vi "Measurement.vi"(1 "setup":T3=enum."Show Setup", 2 "Post Process":T2, 4 "File":T4, 5 "Results file":path, 7 "Raw data file":path, 11 "Setup filename":string) -> (14 "2nd plot":cluster{"X array":dbl[], "Y array":dbl[]}[](graph), 19 "Status Out":T1)   [LabVIEW 2022 SP3]
uses:
  Anemometry Sub Vis/Globals/Meas_global.vi
  Anemometry Sub Vis/Globals/LDA_meas_global_1.vi
  Anemometry Sub Vis/Globals/Dynamic_call_global.ph.vi
  Anemometry Sub Vis/Controls/Post_Process.ctl
  Anemometry Sub Vis/Controls/Setup.ctl
  Anemometry Sub Vis/Gen Trav/Multi_Run_Status.ctl
  Anemometry Sub Vis/Globals/Trav_pos_global.vi
  Anemometry Sub Vis/Controls/Save_Data.ctl
  Anemometry Sub Vis/Acquisition/PWA/PWAtasksGLOBAL.vi
  Anemometry Sub Vis/Globals/Plug_in_data_global.vi
  Anemometry Sub Vis/Controls/Graph_Type.ctl
  ADAM Client/Sub VIs/ADAM Controls/Traverse_Level_State.ctl
  Anemometry Sub Vis/Globals/Preference_global.vi
  Anemometry Sub Vis/File/Setup_Filetype.ctl
  Anemometry Sub Vis/Controls/Inst_type.ctl
  Anemometry Sub Vis/Globals/Constants_global.vi
  Anemometry Sub Vis/Globals/Gas_management_global.vi
  Anemometry Sub Vis/Controls/Time_Trace_Cluster.ctl
  Anemometry Sub Vis/Controls/Instrument_Array.ctl
  <vilib>/Utility/miscctls.llb/LVRowAndColumnTypeDef.ctl
  Anemometry Sub Vis/Globals/LDA_global.vi
  Anemometry Sub Vis/File/File Update Cluster.ctl
  Anemometry Sub Vis/Globals/Extra_Commands_Global.vi
  Anemometry Sub Vis/CTA/CTA Calib Coeff Global.vi
  Anemometry Sub Vis/CTA/Ctls/Calibration data.ctl
panel:
  in  "PP next block":bool
  out "Pause message":string
  out "Statistics":string[][](table)
  in  "Time per Block (s)":dbl=100.0 format="%#_5f"
  out "Current Block No":i32=5 caption="Current Block"
  in  "Pause":bool
  in  "No of Blocks":i32=5
  in  "stop":bool
  out "progress":dbl(slide) scale=0.0..1.0
  in  "Tab Control":T5(tab)
  in  "Second Graph":T7={"Plot 1"=2, "Plot 2"=1, "Save graph"=0, "Plot Type"=enum."Vel histogram"} {"Save graph" items=["Do not save plot", "Save plot"]; "Plot 2" items=["Nothing", "FID4"]; "Plot 1" items=["Nothing", "FID4"]}
  in  "First Graph":T7={"Plot 1"=1, "Plot 2"=2, "Save graph"=0, "Plot Type"=enum."Velocity trace"} {"Save graph" items=["Do not save plot", "Save plot"]; "Plot 2" items=["Nothing", "FID4"]; "Plot 1" items=["Nothing", "FID4"]}
  out "First plot":cluster{"X array":dbl[], "Y array":dbl[]}[](graph)
  in  "Comments":string
  out "uv":dbl[][](graph)=[[-0.041806189081711534, -0.046435429052714985, -0.04035660097427599, -0.042187605126076694, -0.042052555599004206]]
  out "u^4":dbl[][](graph)
  out "u^3":dbl[][](graph)
  out "u^2":dbl[][](graph)=[[0.09743628875280319, 0.10575821456272283, 0.10126262927293661, 0.09890442087602569, 0.1022948212436432]]
  out "U":dbl[][](graph)=[[0.8295029456391334, 0.8915896983798417, 0.8415763502225625, 0.8394746126219594, 0.8466062785395404]]
  in  "Block average display control":cluster{"Name":string, "Include":bool}[](array[cluster])=[{"Name"="FF (C)", "Include"=FALSE}]
  out "blockDone":bool
  in  "Select Duplicate Channels":bool
  in  "Sub Block Time (s) for Spectra and Auto Corr":dbl=1.0 min=1.0 step=1.0
  in  "No of bins in histogram":i32=100
  out "Measurement time (min)":dbl=6.0 format="%.2f"
  in  "Correlate?":T8(ring)
  out "Diagnostic info":string[][](table)
  in  "No of estimates output for when saving plots":i32=200
  out "Position":T9(array[cluster]) {"Z" format="%.1f"; "Y" format="%.1f"; "X" format="%.1f"}
  out "Array U":dbl[][](array[numeric]) format="%.2e"
  out "Array u^2":dbl[][](array[numeric]) format="%.2e"
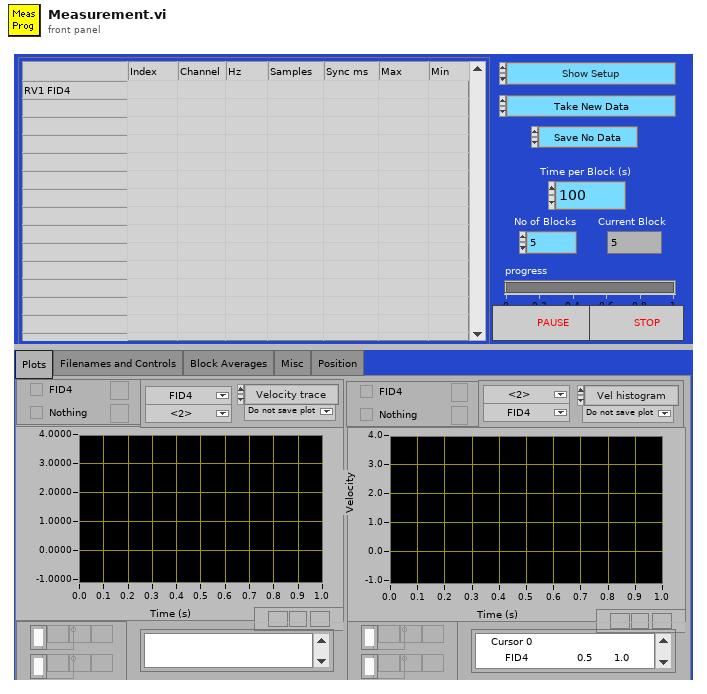
[diagram p1: front panel]
types:
  T1 = typedef "Multi_Run_Status.ctl" = enum16{"Continue", "Continue with Error", "Jump to Next Point", "Jump to Next Row", "Jump To Fall Back", "Terminate Run"}
  T2 = typedef "Post_Process.ctl" = enum16{"Take New Data", "Post Process Raw Data File"}
  T3 = typedef "Setup.ctl" = enum16{"Run Program", "Show Setup", "Save Current Setup", "Setup Front Panel"}
  T4 = typedef "Save_Data.ctl" = enum16{"Save No Data", "Save Data"}
  T5 = enum32{"Plots", "Filenames and Controls", "Block Averages", "Misc", "Position"}
  T6 = typedef "Graph_Type.ctl" = enum16{"Show no graph", "Voltage trace", "Velocity trace", "Vel histogram", "Spectrum", "f.E(f) v Log f", "Auto-Corr"}
  T7 = cluster{"Plot 1":u16, "Plot 2":u16, "Save graph":u16, "Plot Type":T6}
  T8 = enum16{"Cross correlation off", "Show correlation panel", "Correlate without activating panel"}
  T9 = cluster{"Name":string, "X":dbl, "Y":dbl, "Z":dbl}[]
  T10 = typedef "Calibration data.ctl" = cluster{"X cal.[]":dbl[], "Re cal.[]":dbl[], "a1[]":dbl[], "a2[]":dbl[], "a3[]":dbl[]}
  T11 = enum32{"Bad", "Idle", "Run top level", "Running"}
  T12 = typedef "Inst_type.ctl" = enum16{"Raw voltage", "Raw with zero offsetting", "Propeller anemometer", "Pressure Transducer", "Pitot-static tube", "Hot wire", "Cross wire 1", "Cross wire 2", "Generic Linear", "Generic Polynomial", "Generic BackPoly", "Fast FID", "Thermocouple", "Cold wire", "Pulsed Wire", "LDA Vel", "LDA Tran time", "LDA Arr time", "Microphone"}
  T13 = cluster{"Name":string, "X":dbl, "Y":dbl, "Z":dbl}
  T14 = enum32{"Invalid", "Standard", "Closed", "Hidden", "Minimized", "Maximized"}
  T15 = enum16{"Save no data", "Save data in new files", "Save data in existing files"}
  T16 = typedef "Time_Trace_Cluster.ctl" = cluster{"Weighting":dbl[], "Voltage":dbl[], "Eng Values":dbl[]}
  T17 = enum16{"Zero or one", "One", "Zero or more", "One or more"}
  T18 = typedef "Traverse_Level_State.ctl" = enum16{"Running", "Complete"}
  T19 = typedef "LVRowAndColumnTypeDef.ctl" = cluster{"Row":i32, "Column":i32}
  T20 = typedef "Instrument_Array.ctl" = enum16{"PWA", "LDA", "Analogue"}
  T21 = typedef "Setup_Filetype.ctl" = enum16{"Measurement Setups", "Calibration Setups", "General", "Results File Plotter Setups", "Speed Calib Tweaks"}
  T22 = typedef "File Update Cluster.ctl" = cluster{"File Path":path, "Rows to Add":i32[], "Extra Ch Names":string[], "Extra Ch Values":string[], "Initial Header String":string, "Separation Character":enum16{"Tab", "Comma"}}
  T23 = typedef "Analysis_info_cluster.ctl" = cluster{"Colour":u32, "Inst type":T12, "Inst name":string, "Symbol":string, "Code name":string, "Extra Info":string, "Inst Array":T20, "U":dbl, "u^2":dbl, "u^3":dbl, "u^4":dbl, "Skew_u":dbl, "Kurt_u":dbl, "Sd Error in Mean":dbl, "% u'/U":dbl, "X":dbl, "Y":dbl, "Z":dbl, "Timescale integral Estimate":dbl, "Sd Error in Variance":dbl, "Calib File":path, "Calib Constants":dbl[], "Output Position":bool, "Stats":enum16{"None", "Basic", "Full"}, "Av Sampling Rate":dbl, "Av No of Samples":dbl, "Total Meas Time (s)":dbl, "OrigChName":string, "Max value":dbl, "Min value":dbl, "Req Sample Rate Hz":dbl, "Sync Delay Time (s)":dbl, "Ch No":i16, "Device":string, "Use Latest Calib":bool, "Port":string, "Metadata Ch Names":string[], "Metadata Ch Values":string[], "Label":string, "chState":T24, "Point Drift":dbl, "inputConfig":string}
  T24 = typedef "channelState.ctl" = enum32{"No Selection", "Solo", "Mute"}
  T25 = cluster{"Insts for plotting[0]":u16, "Insts for plotting[1]":u16}
  T26 = typedef "Device ID port info.ctl" = cluster{"Ch No":i16[], "Req Sampling Rate":dbl[], "Port":string, "Index":i32[]}
  T27 = typedef "Rendezvous RefNum" = refnum<k1>
  T28 = typedef "PWA_Data.ctl" = enum16{"No PWA Data", "One Ch PWA"}
  T29 = typedef "LDA_Channel.ctl" = cluster{"Wavelength (nm)":dbl, "Vel Comp":string, "Max Velocity":dbl, "Min Velocity":dbl, "Max Record length":u16, "Signal gain (dB)":i16, "High voltage":i16, "Optics Conversion Factor":dbl, "Min Record length":u16, "Multiply Velocity by -1":bool, "Signal to Noise Ratio":string, "Validation Ratio":string, "Probe":string, "Laser":string, "BSA":string, "Lense":string, "Beam Separation (mm)":dbl, "Focal Length (mm)":dbl, "COLOUR":u32, "BSA IP":string, "Velocity Range (m/s)":dbl, "Centre Velocity (m/s)":dbl, "Unshifted mW":dbl, "Shifted mW":dbl, "Bandwidth Hz":dbl, "Req Sampling Rate Hz":dbl, "Ch":i32, "CenterFreq Hz":dbl, "Laser IP":string, "Sync Delay (s)":dbl}
  T30 = typedef "Correlation_cluster1.ctl" = cluster{"U inst":string, "uw":dbl, "u^2w":dbl, "uw^2":dbl, "uw/u'w'":dbl, "W inst":string, "uw^3":dbl, "u^3w":dbl, "u^2w^2":dbl, "Index U":i32, "Index W":i32, "Error info":string[], "Paired Sampling Rate (Hz)":dbl, "u^2 Paired":dbl, "w^2 Paired":dbl, "Time Window (ms)":dbl}
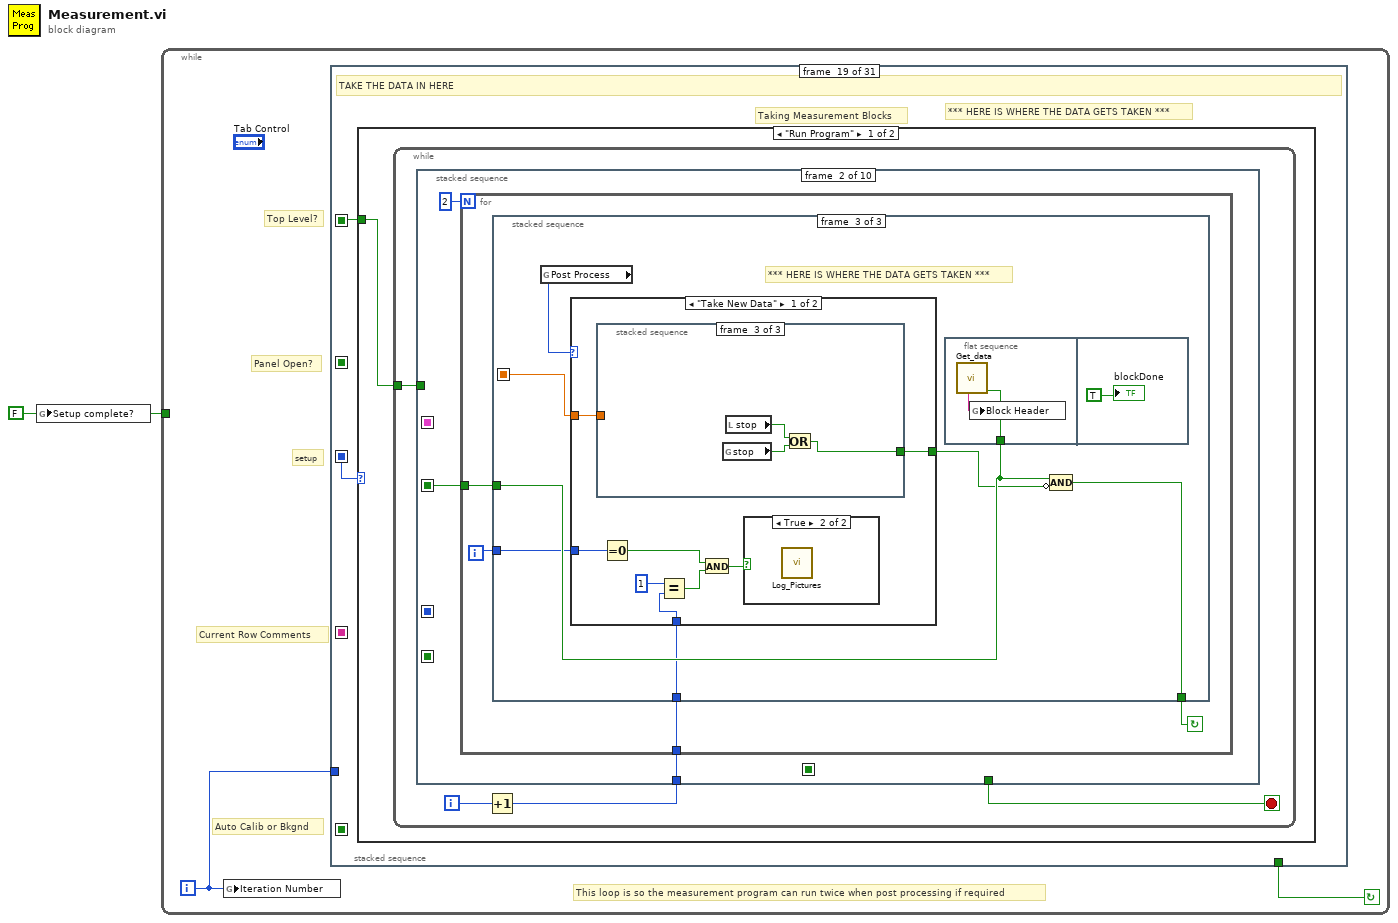
[diagram p0: block diagram]
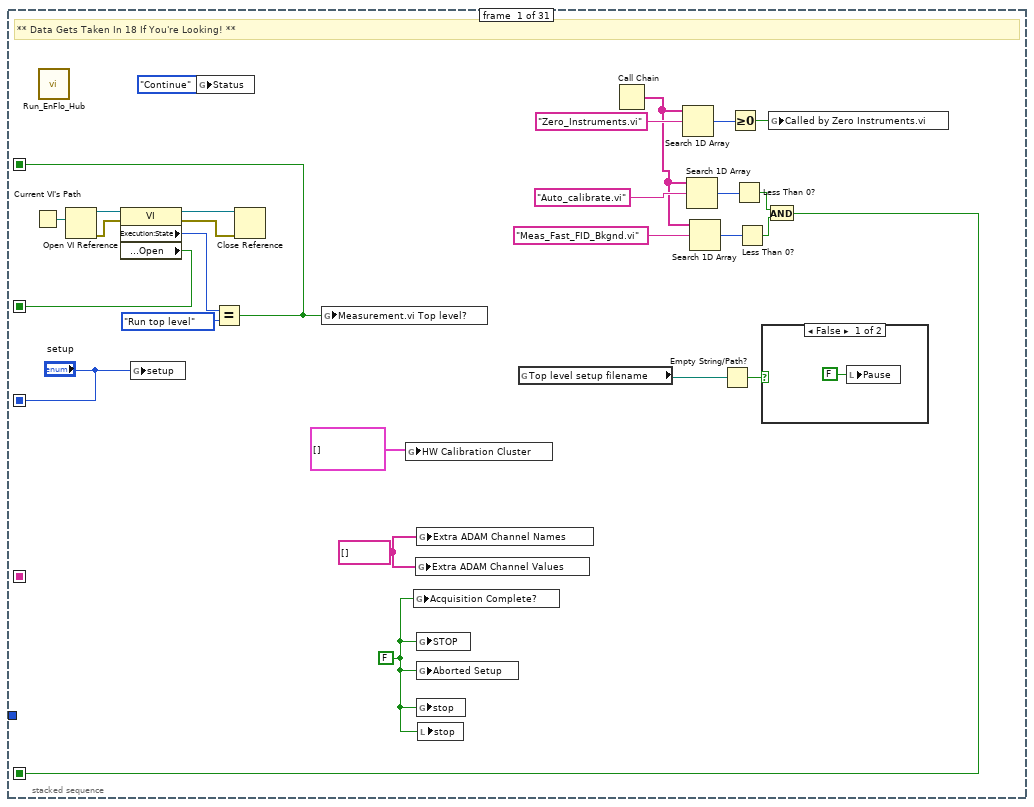
[diagram p2: hidden frame]
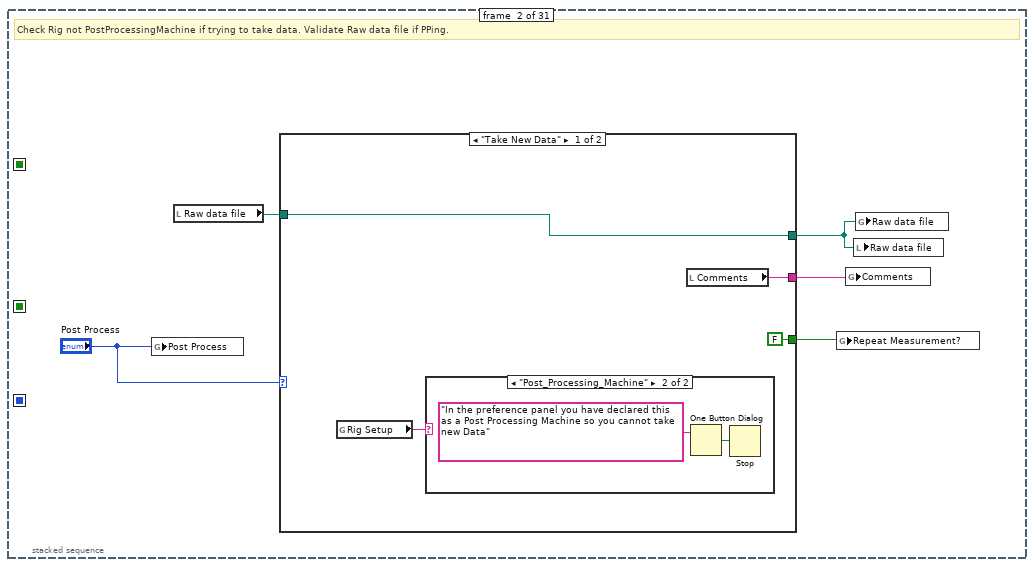
[diagram p4: hidden frame]
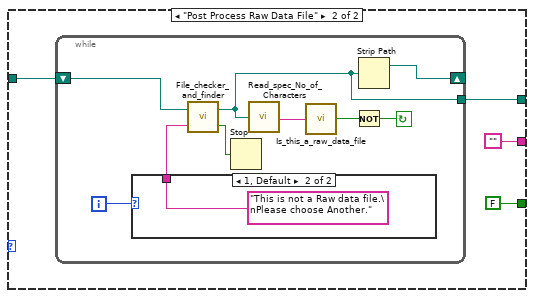
[diagram p6: hidden frame]
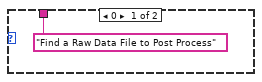
[diagram p7: hidden frame]
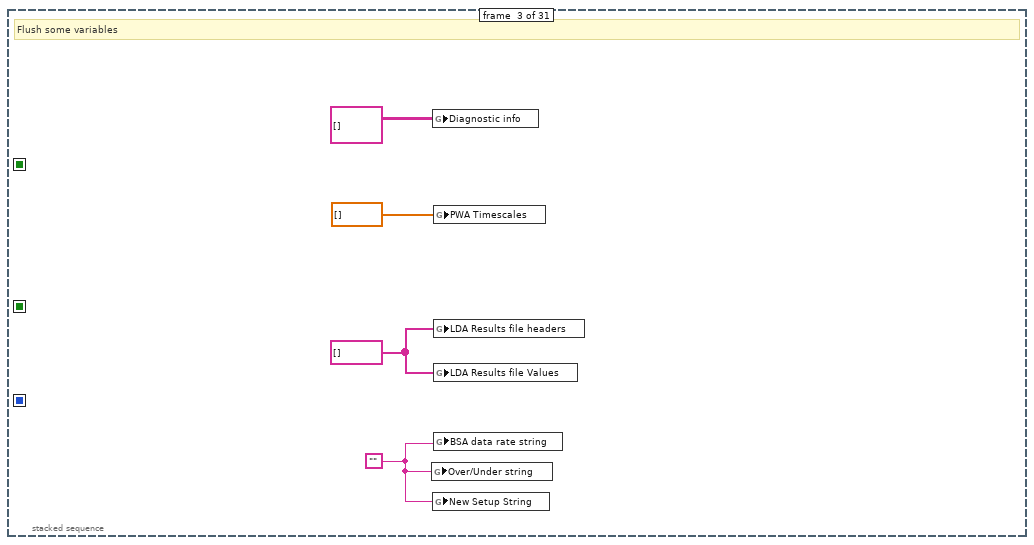
[diagram p8: hidden frame]
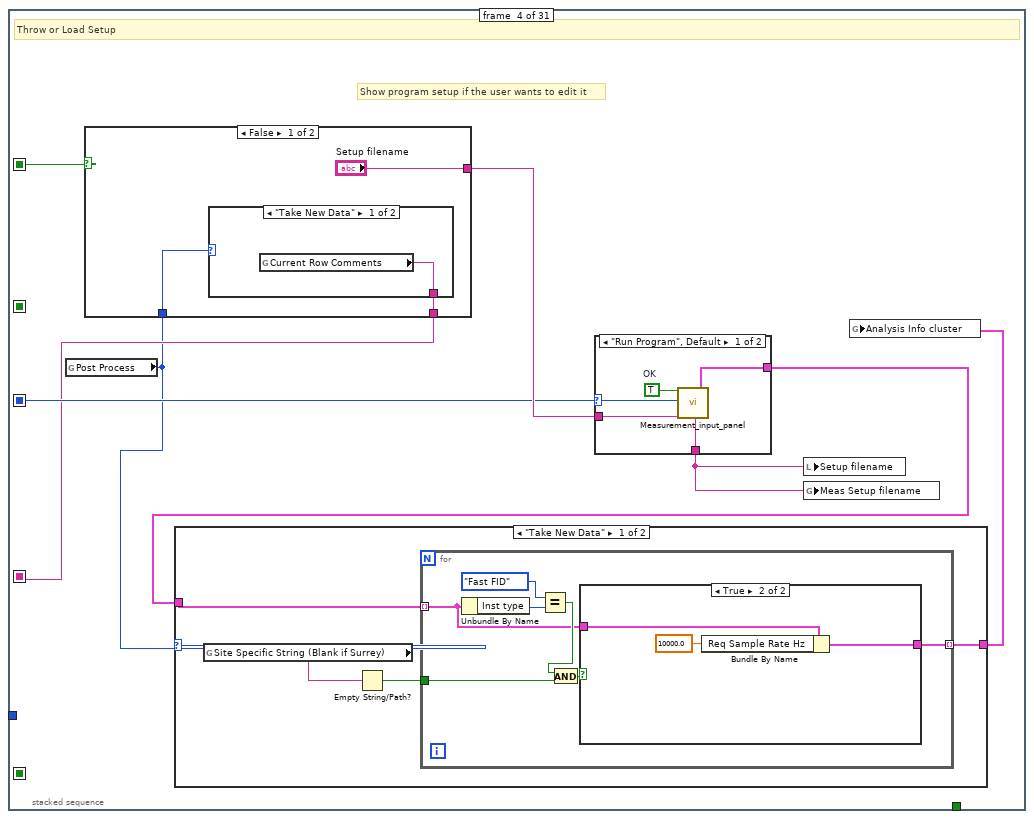
[diagram p9: hidden frame]
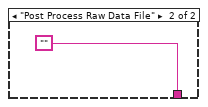
[diagram p12: hidden frame]
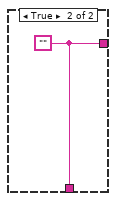
[diagram p13: hidden frame]
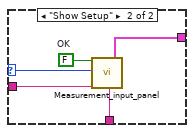
[diagram p14: hidden frame]
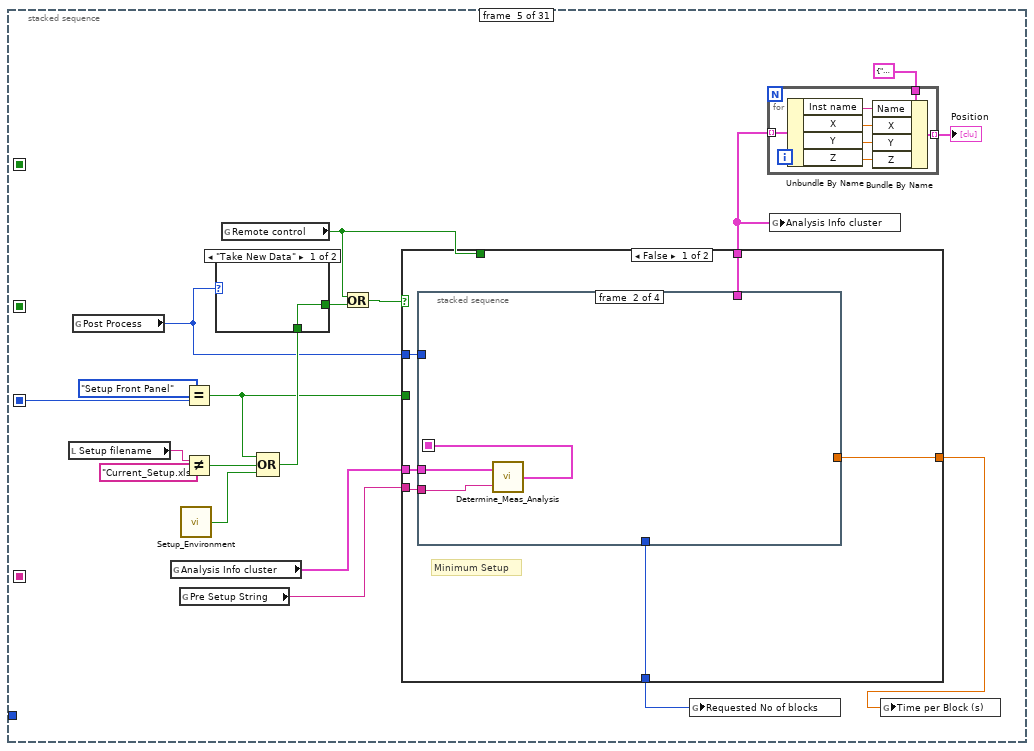
[diagram p15: hidden frame]
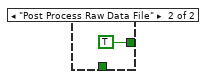
[diagram p16: hidden frame]
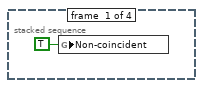
[diagram p17: hidden frame]
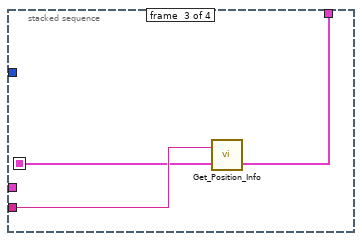
[diagram p18: hidden frame]
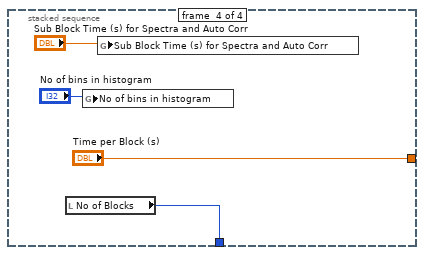
[diagram p19: hidden frame]
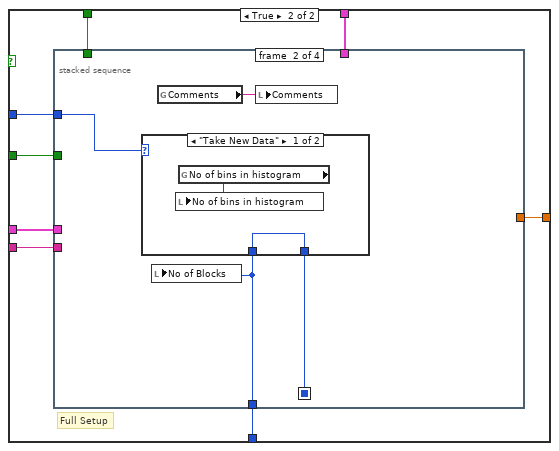
[diagram p20: hidden frame]
diagram:
  w1 = FALSE ("Setup complete?")
  n1 = global write "Meas_global.vi" "Setup complete?"(w1) -> ()
  n2 = while {
    tunnel: w1 -> [_]
    i -> [w2]
    stop <- w3 continue-if-true
    # "Auto Calib or Bkgnd"
    # "Current Row Comments"
    # "This loop is so the measurement program can run twice when post processing if required"
    # "Panel Open?"
    # "Top Level?"
    # "setup"
    n3 = global write "Meas_global.vi" "Iteration Number"(w2) -> ()
    n4 = stacked-sequence {
      seq-local: ["setup" _ _ _ _ _ _ _ _ _ _ _ _ _ _ _ _ _ _ _ _ _ _ _ _ _ _ _ _ _ _] -> [_ _ _ w67 w113 _ _ _ w235 _ w299 _ _ w538 _ w721 w749 _ w763 w1064 _ _ w1200 w1229 w1278 w1307 w1368 w1451 _ _ _]
      seq-local: [w15 _ _ _ _ _ _ _ _ _ _ _ _ _ _ _ _ _ _ _ _ _ _ _ _ _ _ _ _ _ _] -> [_ _ _ w66 _ _ _ _ _ _ w275 _ _ _ _ w719 _ _ w762 _ _ _ _ _ _ _ _ _ _ _ _]
      seq-local: [w23 _ _ _ _ _ _ _ _ _ _ _ _ _ _ _ _ _ _ _ _ _ _ _ _ _ _ _ _ _ _] -> [_ _ _ _ _ _ _ _ _ _ _ _ _ w539 _ _ _ _ _ _ _ _ _ _ _ _ _ _ _ _ _]
      seq-local: [_ _ _ w65 _ _ _ _ _ _ _ _ _ _ _ _ _ _ _ _ _ _ _ _ _ _ _ _ _ _ _] -> [_ _ _ _ _ _ _ _ _ w270 _ _ _ _ _ _ _ _ _ _ _ _ _ _ _ _ _ _ w1468 _ _]
      seq-local: [w4 _ _ _ _ _ _ _ _ _ _ _ _ _ _ _ _ _ _ _ _ _ _ _ _ _ _ _ _ _ _] -> [_ _ _ _ _ _ _ _ _ _ _ _ _ _ _ _ _ _ _ _ _ _ _ w1225 _ _ _ _ _ _ _]
      tunnel: w2 -> [_ _ _ _ _ _ _ _ _ _ _ _ _ _ _ _ _ _ _ _ _ _ _ _ _ _ _ _ w1477 _ _]
      tunnel: [_ _ _ _ _ _ _ _ _ _ _ _ _ _ _ _ _ _ _ _ _ _ _ _ _ _ _ _ w1476 _ _] -> w3
      frame #0 {
        w20 = string[] [] ("Extra ADAM Channel Names")
        w13 = FALSE ("Processing last block?")
        # "** Data Gets Taken In 18 If You're Looking! **"
        n5 = Current VI's Path() -> (path=w24:path)
        n6 = call "Run_EnFlo_Hub.vi"() -> ()  [unwired: 1 in, 7 out]
        n7 = Open VI Reference(vi path=w24) -> (vi reference=w25:refnum<vi>, error out=w26:errorcluster)  [unwired: 1 in, 4 out]
        n8 = property class="VI"(reference=w25, error in=w26) -> (reference out=w27:refnum<vi>, error out=w28:errorcluster, "Execution:State"=w29:T11, "Front Panel.Open"=w23:bool)
        n9 = global write "Meas_global.vi" "setup"("setup") -> ()
        n10 = global write "Meas_global.vi" "Status"(Multi_Run_Status."Continue" ("Status")) -> ()
        n11 = Equal?(x=w29, y=T11."Run top level" ("Exec.State")) -> (x = y?=w15:bool)
        n12 = Close Reference(reference=w27, error in (no error)=w28) -> ()  [unwired: 1 out]
        n13 = global write "Meas_global.vi" "Measurement.vi Top level?"(w15) -> ()
        n14 = global write "CTA Calib Coeff Global.vi" "HW Calibration Cluster"(T10[] [] ("HW Calibration Cluster")) -> ()
        n15 = global write "Meas_global.vi" "Acquisition Complete?"(w13) -> ()
        n16 = global write "Meas_global.vi" "Extra ADAM Channel Values"(w20) -> ()
        n17 = global write "Meas_global.vi" "Extra ADAM Channel Names"(w20) -> ()
        n18 = global write "PWAtasksGLOBAL.vi" "STOP"(w13) -> ()
        n19 = global write "Meas_global.vi" "Aborted Setup"(w13) -> ()
        n20 = global write "Meas_global.vi" "stop"(w13) -> ()
        n21 = local write "stop"(w13) -> ()
        n22 = global read "Trav_pos_global.vi" "Top level setup filename"() -> (w22:path)
        n23 = Call Chain() -> (call chain=w9:string[])
        n24 = Search 1D Array(1D array=w9, element="Zero_Instruments.vi") -> (index of element=w18:i32)  [unwired: 1 in]
        n25 = Search 1D Array(1D array=w9, element="Auto_calibrate.vi") -> (index of element=w11:i32)  [unwired: 1 in]
        n26 = Search 1D Array(1D array=w9, element="Meas_Fast_FID_Bkgnd.vi") -> (index of element=w7:i32)  [unwired: 1 in]
        n27 = Empty String/Path?(string/path=w22) -> (empty?=w21:bool)
        n28 = Greater Or Equal To 0?(x=w18) -> (x >= 0?=w17:bool)
        n29 = Less Than 0?(x=w11) -> (x < 0?=w5:bool)
        n30 = Less Than 0?(x=w7) -> (x < 0?=w6:bool)
        n31 = case shown="False" w21 {
          frame False {
            n32 = local write "Pause"(FALSE ("Pause")) -> ()
          }
          frame True {
          }
        }
        n33 = And(x=w5, y=w6) -> (x .and. y?=w4:bool)
        n34 = global write "Meas_global.vi" "Called by Zero Instruments.vi"(w17) -> ()
      }
      frame #1 {
        # "Check Rig not PostProcessingMachine if trying to take data. Validate Raw data file if PPing."
        n35 = global write "Meas_global.vi" "Post Process"("Post Process") -> ()
        n36 = local read "Raw data file"() -> (w36:path)
        n37 = case shown="\"Take New Data\"" "Post Process" {
          tunnel: [w40 w46] -> w35
          tunnel: w36 -> [w40 w45]
          tunnel: [FALSE FALSE] -> w33
          tunnel: [w38 ""] -> w32
          frame "Take New Data" {
            n38 = global read "Preference_global.vi" "Rig Setup"() -> (w37:string)
            n39 = case shown="\"Post_Processing_Machine\"" w37 {
              frame "False", Default {
              }
              frame "Post_Processing_Machine" {
                n40 = One Button Dialog(message="In the preference panel you have declared this as a Post Processing Machine so you cannot take new Data") -> (true=w41:bool)  [unwired: 1 in]
                n41 = Stop(stop? (T)=w41) -> ()
              }
            }
            n42 = local read "Comments"() -> (w38:string)
          }
          frame "Post Process Raw Data File" {
            n43 = while {
              tunnel: [w48] -> w46
              shift-left: w45 -> [w50]
              shift-right: [w49] -> _
              i -> [w51]
              stop <- w52 continue-if-true
              n44 = case shown="1, Default" w51 {
                tunnel: ["Find a Raw Data File to Post Process" ("Promp if not found") "This is not a Raw data file.\nPlease choose Another." ("Promp if not found")] -> w55
                frame 0 {
                }
                frame 1, Default {
                }
              }
              n45 = call "File_checker_and_finder.vi"("Promp if not found"=w55, "Filename In"=w50) -> ("cancelled"=w47:bool, "Filename Out"=w48:path)
              n46 = Stop(stop? (T)=w47) -> ()
              n47 = call "Read_spec_No_of_Characters.vi"("Filename"=w48) -> ("character string"=w54:string)  [unwired: 1 out]
              n48 = call "Is_this_a_raw_data_file.vi"("character string"=w54) -> ("Raw Dat File?"=w53:bool)  [unwired: 2 out]
              n49 = Not(x=w53) -> (.not. x?=w52:bool)
              n50 = Strip Path(path=w48) -> (stripped path=w49:path)  [unwired: 1 out]
            }
          }
        }
        n51 = global write "Meas_global.vi" "Repeat Measurement?"(w33) -> ()
        n52 = global write "Meas_global.vi" "Comments"(w32) -> ()
        n53 = local write "Raw data file"(w35) -> ()
        n54 = global write "Meas_global.vi" "Raw data file"(w35) -> ()
      }
      frame #2 {
        w60 = string[] [] ("Plug in values")
        w61 = ""
        # "Flush some variables"
        n55 = global write "Meas_global.vi" "Over/Under string"(w61) -> ()
        n56 = global write "Meas_global.vi" "Diagnostic info"(string[][] [] ("Diagnostic info")) -> ()
        n57 = global write "Meas_global.vi" "New Setup String"(w61) -> ()
        n58 = global write "PWAtasksGLOBAL.vi" "PWA Timescales"(dbl[] [] ("LDA Timescales")) -> ()
        n59 = global write "LDA_meas_global_1.vi" "LDA Results file headers"(w60) -> ()
        n60 = global write "LDA_meas_global_1.vi" "LDA Results file Values"(w60) -> ()
        n61 = global write "Meas_global.vi" "BSA data rate string"(w61) -> ()
      }
      frame #3 {
        # "Show program setup if the user wants to edit it"
        # "Throw or Load Setup"
        n62 = global read "Meas_global.vi" "Post Process"() -> (w64:T2)
        n63 = case shown="False" w66 {
          tunnel: ["Setup filename" w91] -> w69
          tunnel: [w87 w91] -> w65
          tunnel: w64 -> [w86 _]
          frame False {
            n64 = case shown="\"Take New Data\"" w86 {
              tunnel: [w89 ""] -> w87
              frame "Take New Data" {
                n65 = global read "Meas_global.vi" "Current Row Comments"() -> (w89:string)
              }
              frame "Post Process Raw Data File" {
              }
            }
          }
          frame True {
            w91 = ""
          }
        }
        n66 = case shown="\"Run Program\", Default" w67 {
          selector: w67 -> [w92 w97]
          tunnel: [w95 w100] -> w63
          tunnel: w69 -> [w94 w99]
          tunnel: [w93 w98] -> w68
          frame "Run Program", Default {
            w96 = TRUE  # OK
            n67 = call "Measurement_input_panel.vi"("OK"=w96, "setup"=w92, "Setup filename"=w94) -> ("Setup filename out"=w93:string, "Analysis Info cluster"=w95:T23[])  [unwired: 15 out]
          }
          frame "Show Setup" {
            w101 = FALSE  # OK
            n68 = call "Measurement_input_panel.vi"("OK"=w101, "setup"=w97, "Setup filename"=w99) -> ("Setup filename out"=w98:string, "Analysis Info cluster"=w100:T23[])  [unwired: 15 out]
          }
        }
        n69 = case shown="\"Take New Data\"" w64 {
          tunnel: w63 -> [w73 w85]
          tunnel: [w70 w85] -> w62
          frame "Take New Data" {
            n70 = global read "Preference_global.vi" "Site Specific String (Blank if Surrey)"() -> (w72:string)
            n71 = Empty String/Path?(string/path=w72) -> (empty?=w71:bool)
            n72 = for {
              tunnel: w73 -> [w75] mode=indexing
              tunnel: w71 -> [w76]
              tunnel: [w74] -> w70 mode=indexing
              n73 = Unbundle By Name(w75) -> ("Inst type"=w79:T12)
              n74 = Equal?(x=Inst_type."Fast FID" ("Inst type"), y=w79) -> (x = y?=w77:bool)
              n75 = And(x=w77, y=w76) -> (x .and. y?=w78:bool)
              n76 = case shown="True" w78 {
                tunnel: w75 -> [w81 w84]
                tunnel: [w81 w82] -> w74
                frame False {
                }
                frame True {
                  n77 = Bundle By Name(cluster=w84, "Req Sample Rate Hz"=10000.0) -> (w82:T23)
                }
              }
            }
          }
          frame "Post Process Raw Data File" {
          }
        }
        n78 = local write "Setup filename"(w68) -> ()
        n79 = global write "Meas_global.vi" "Meas Setup filename"(w68) -> ()
        n80 = global write "Meas_global.vi" "Analysis Info cluster"(w62) -> ()
      }
      frame #4 {
        n81 = local read "Setup filename"() -> (w117:string)
        n82 = global read "Meas_global.vi" "Post Process"() -> (w112:T2)
        n83 = global read "Meas_global.vi" "Analysis Info cluster"() -> (w105:T23[])
        n84 = global read "Meas_global.vi" "Pre Setup String"() -> (w108:string)
        n85 = call "Setup_Environment.vi"() -> ("First Time"=w109:bool)  [unwired: 1 in]
        n86 = Equal?(x=Setup."Setup Front Panel" ("setup"), y=w113) -> (x = y?=w106:bool)
        n87 = Not Equal?(x=w117, y="Current_Setup.xls" ("Setup filename")) -> (x != y?=w115:bool)
        n88 = global read "Meas_global.vi" "Remote control"() -> (w107:bool)
        n89 = Compound Arithmetic op=OR(w106, w115, w109) -> (w114:bool)
        n90 = case shown="\"Take New Data\"" w112 {
          tunnel: [w128 TRUE] -> w120
          tunnel: w114 -> [w128 _]
          frame "Take New Data" {
          }
          frame "Post Process Raw Data File" {
          }
        }
        n91 = Or(x=w107, y=w120) -> (x .or. y?=w119:bool)
        n92 = case shown="False" w119 {
          tunnel: w112 -> [w132 w154]
          tunnel: [w135 w153] -> w110
          tunnel: [w134 w149] -> w118
          tunnel: [w133 w152] -> w104
          tunnel: w108 -> [w131 w151]
          tunnel: w107 -> [_ w150]
          tunnel: w106 -> [_ w148]
          tunnel: w105 -> [w130 w147]
          frame False {
            # "Minimum Setup"
            n93 = stacked-sequence {
              seq-local: [_ w138 _ _] -> [_ _ w140 _]
              tunnel: [_ _ _ "Time per Block (s)"] -> w135
              tunnel: [_ _ _ w145] -> w134
              tunnel: [_ _ w142 _] -> w133
              tunnel: w132 -> [_ _ _ _]
              tunnel: w131 -> [_ w137 w141 _]
              tunnel: w130 -> [_ w139 _ _]
              frame #0 {
                n94 = global write "LDA_global.vi" "Non-coincident"(TRUE ("Non-coincident")) -> ()
              }
              frame #1 {
                n95 = call "Determine_Meas_Analysis.vi"("Pre Setup String"=w137, "Analysis info Cluster In"=w139) -> ("Analysis info Cluster Out"=w138:T23[])
              }
              frame #2 {
                n96 = call "Get_Position_Info.vi"("Analysis Info cluster"=w140, "Setup file string"=w141) -> ("Analysis Info cluster 2"=w142:T23[])  [unwired: 1 in]
              }
              frame #3 {
                n97 = local read "No of Blocks"() -> (w145:i32)
                n98 = global write "Meas_global.vi" "No of bins in histogram"("No of bins in histogram") -> ()
                n99 = global write "Meas_global.vi" "Sub Block Time (s) for Spectra and Auto Corr"("Sub Block Time (s) for Spectra and Auto Corr") -> ()
              }
            }
          }
          frame True {
            # "Full Setup"
            n100 = stacked-sequence {
              seq-local: [w157 _ _ _] -> [_ w161 _ _]
              tunnel: w154 -> [_ w162 _ w178]
              tunnel: [w159 _ _ _] -> w153
              tunnel: [w156 _ _ _] -> w152
              tunnel: w151 -> [w158 _ _ _]
              tunnel: w150 -> [_ _ w170 _]
              tunnel: [_ w160 _ _] -> w149
              tunnel: w148 -> [_ _ w169 _]
              tunnel: w147 -> [w155 _ _ _]
              frame #0 {
                n101 = call "Read_raw_meas_setup.vi"("Setup file string"=w158, "Analysis Info cluster In"=w155) -> ("No of Blocks"=w157:i32, "Time per Block (s)"=w159:dbl, "Analysis Info clusterOut"=w156:T23[])  [unwired: 5 out]
                n102 = local write "Time per Block (s)"(w159) -> ()
              }
              frame #1 {
                n103 = case shown="\"Take New Data\"" w162 {
                  tunnel: [w165 99999 ("No of Blocks")] -> w160
                  tunnel: w161 -> [w165 _]
                  frame "Take New Data" {
                    n104 = global read "Meas_global.vi" "No of bins in histogram"() -> (w164:i32)
                    n105 = local write "No of bins in histogram"(w164) -> ()
                  }
                  frame "Post Process Raw Data File" {
                    n106 = local read "No of bins in histogram"() -> (w166:i32)
                    n107 = global write "Meas_global.vi" "No of bins in histogram"(w166) -> ()
                  }
                }
                n108 = local write "No of Blocks"(w160) -> ()
                n109 = global read "Meas_global.vi" "Comments"() -> (w163:string)
                n110 = local write "Comments"(w163) -> ()
              }
              frame #2 {
                n111 = Or(x=w170, y=w169) -> (x .or. y?=w168:bool)
                n112 = case shown="True" w168 {
                  frame False {
                  }
                  frame True {
                    n113 = global read "Meas_global.vi" "Pre Setup String"() -> (w171:string)
                    n114 = call "Get_Characters_from_string.vi"("Input string"=w171, "Variable name"="Results filename") -> ("Status"=w174:enum16{"Char in string", "Char not in string"}, "Value"=w173:string)  [unwired: 1 in]
                    n115 = case shown="\"Char in string\"" w174 {
                      tunnel: w173 -> [w176 _]
                      frame "Char in string" {
                        n116 = String To Path(string=w176) -> (path=w175:path)
                        n117 = local write "Results file"(w175) -> ()
                      }
                      frame "Char not in string" {
                      }
                    }
                  }
                }
              }
              frame #3 {
                n118 = global read "Meas_global.vi" "Sub Block Time (s) for Spectra and Auto Corr"() -> (w177:dbl)
                n119 = case shown="\"Take New Data\"" w178 {
                  frame "Take New Data" {
                    n120 = global read "Meas_global.vi" "Second Graph"() -> (w179:T7)
                    n121 = global read "Meas_global.vi" "First Graph"() -> (w180:T7)
                    n122 = local write "Second Graph"(w179) -> ()
                    n123 = local write "First Graph"(w180) -> ()
                  }
                  frame "Post Process Raw Data File" {
                  }
                }
                n124 = local write "Sub Block Time (s) for Spectra and Auto Corr"(w177) -> ()
              }
            }
          }
        }
        n125 = global write "Meas_global.vi" "Requested No of blocks"(w118) -> ()
        n126 = for {
          tunnel: w104 -> [w127] mode=indexing
          tunnel: [w123] -> w102 mode=indexing
          tunnel: T13 {"Name"="", "X"=0.0, "Y"=0.0, "Z"=0.0} ("Position") -> [w122]
          n127 = Unbundle By Name(w127) -> ("Inst name"=w121:string, "X"=w124:dbl, "Y"=w125:dbl, "Z"=w126:dbl)
          n128 = Bundle By Name(cluster=w122, "Name"=w121, "X"=w124, "Y"=w125, "Z"=w126) -> (w123:T13)
        }
        "Position" <- w102
        n129 = global write "Meas_global.vi" "Analysis Info cluster"(w104) -> ()
        n130 = global write "Meas_global.vi" "Time per Block (s)"(w110) -> ()
      }
      frame #5 {
        # "Launch Initial plugins, if any"
        n131 = global read "Dynamic_call_global.ph.vi" "Initial Plug Ins Extra"() -> (w184:string[])
        n132 = global read "Dynamic_call_global.ph.vi" "Initial Plug Ins"() -> (w183:string[])
        n133 = Build Array (concatenate)(w184, w183) -> (w181:string[])
        n134 = Empty Array?(array=w181) -> (empty?=w182:bool)
        n135 = case shown="False" w182 {
          tunnel: w181 -> [_ w185]
          frame True {
          }
          frame False {
            n136 = stacked-sequence {
              tunnel: w185 -> [w187 _]
              frame #0 {
                n137 = call "Analyse_string_array.vi"("String array"=w187) -> ("Unique strings"=w186:string[])  [unwired: 1 in, 1 out]
                n138 = global read "Meas_global.vi" "Post Process"() -> (w190:T2)
                n139 = call "Plug_in_Directories.vi"() -> ("Initial"=w188:path)  [unwired: 2 in, 4 out]
                n140 = Equal?(x=w190, y=Post_Process."Post Process Raw Data File" ("Post Process")) -> (x = y?=w189:bool)
                n141 = for {
                  tunnel: w189 -> [w202]
                  tunnel: w186 -> [w199] mode=indexing
                  tunnel: w188 -> [w198]
                  w204 = FALSE  # Dialog Box (T)
                  n142 = Build Path(base path=w198, name or relative path=w199) -> (appended path=w200:path)
                  n143 = Open VI Reference(vi path=w200) -> (vi reference=w197:refnum<vi>, error out=w194:errorcluster)  [unwired: 2 in, 3 out]
                  n144 = invoke class="VI" method="FP.Open"(reference=w197, error in=w194, "Activate"=FALSE ("Activate?"), "State"=T14."Standard") -> (reference out=w196:refnum<vi>, error out=w195:errorcluster)  [unwired: 1 in, 3 out]
                  n145 = invoke class="VI" method="Run VI"(reference=w196, error in=w195, "Wait until done"=w202, "Auto Dispose Ref"=FALSE) -> (reference out=w207:refnum<vi>, error out=w206:errorcluster)  [unwired: 1 in, 3 out]
                  n146 = Close Reference(reference=w207, error in (no error)=w206) -> (error out=w205:errorcluster)
                  n147 = call "EnFlo_Error_Handler.vi"("error in (no error)"=w205, "Error Type"="Launching Initial Plug In", "Dialog Box (F)"=w204) -> ()  [unwired: 3 out]
                }
              }
              frame #1 {
                n148 = global read "Meas_global.vi" "Requested No of blocks"() -> (w209:i32)
                n149 = global read "Meas_global.vi" "Comments"() -> (w208:string)
                n150 = local write "Comments"(w208) -> ()
                n151 = local write "No of Blocks"(w209) -> ()
              }
            }
          }
        }
      }
      frame #6 {
        # "Additional Channels"
        n152 = call "Additional Channels.vi"() -> ()  [unwired: 12 in]
      }
      frame #7 {
        # "MeasurementStartTime"
        n153 = global read "Meas_global.vi" "Post Process"() -> (w211:T2)
        n154 = case shown="\"Post Process Raw Data File\"" w211 {
          tunnel: [w213 w214] -> w210
          frame "Take New Data" {
            n155 = Get Date/Time In Seconds() -> (seconds since 1Jan1904=w212:timestamp)
            n156 = To Double Precision Float(number=w212) -> (double precision float=w213:dbl)
          }
          frame "Post Process Raw Data File" {
            n157 = global read "Meas_global.vi" "Pre Setup String"() -> (w217:string)
            n158 = call "Get_Characters_from_string.vi"("Input string"=w217, "Variable name"="Seconds since 1/1/04") -> ("Value"=w215:string)  [unwired: 1 in, 1 out]
            n159 = call "String_2_Number.vi"("Value"=w215) -> ("Numeric"=w214:dbl)
          }
        }
        n160 = global write "Meas_global.vi" "Time Data was Aquired"(w210) -> ()
        n161 = global write "Meas_global.vi" "MeasurementStartTime"(w210) -> ()
      }
      frame #8 {
        # "Establish gas sources"
        n162 = global read "Trav_pos_global.vi" "Source Control?"() -> (w237:bool)
        n163 = global read "Meas_global.vi" "Analysis Info cluster"() -> (w220:T23[])
        n164 = local read "Setup filename"() -> (w228:string)
        n165 = for {
          tunnel: w220 -> [w244] mode=indexing
          tunnel: [w241] -> w219 mode=indexing
          n166 = Unbundle By Name(w244) -> ("Inst type"=w243:T12)
          n167 = Equal?(x=Inst_type."Fast FID" ("Inst type"), y=w243) -> (x = y?=w241:bool)
        }
        n168 = global read "Meas_global.vi" "Post Process"() -> (w226:T2)
        n169 = global read "Preference_global.vi" "Rig Setup"() -> (w223:string)
        n170 = global read "Dynamic_call_global.ph.vi" "Initial Plug Ins"() -> (w240:string[])
        n171 = Equal?(x=w223, y="EnFlo_Tunnel") -> (x = y?=w221:bool)
        n172 = Equal?(x=w226, y=Post_Process."Take New Data" ("Post Process")) -> (x = y?=w224:bool)
        n173 = Equal?(x=Setup."Run Program" ("setup"), y=w235) -> (x = y?=w233:bool)
        n174 = Not Equal?(x=w228, y="Meas_FF_Bkgnd_Setup.xls") -> (x != y?=w232:bool)
        n175 = Not Equal?(x=w228, y="Auto_Calib_Setup.xls") -> (x != y?=w227:bool)
        n176 = Search 1D Array(1D array=w240, element="Puff_using_Arduino.vi") -> (index of element=w238:i32)  [unwired: 1 in]
        n177 = Or Array Elements(Boolean array=w219) -> (logical OR=w218:bool)
        n178 = Less Than 0?(x=w238) -> (x < 0?=w230:bool)
        n179 = Compound Arithmetic op=AND(w237, w233, w232, w227, w224, w221, w218) -> (w231:bool)
        n180 = case shown="True" w231 {
          tunnel: w230 -> [_ w245]
          frame False {
          }
          frame True {
            n181 = global read "Gas_management_global.vi" "Source Live"() -> (w246:bool)
            n182 = Not(x=w246) -> (.not. x?=w247:bool)
            n183 = Select(t=w246, s=w245, f=w247) -> (s? t:f=w248:bool)
            n184 = global read "Preference_global.vi" "Default Source Establishment Time (s)"() -> (w249:dbl)
            n185 = case shown="False" w248 {
              tunnel: w249 -> [w251 w264]
              tunnel: w245 -> [w250 _]
              frame False {
                n186 = stacked-sequence {
                  tunnel: w251 -> [_ w260]
                  tunnel: w250 -> [w252 _]
                  frame #0 {
                    n187 = case shown="False" w252 {
                      tunnel: [w257 w259] -> w254
                      tunnel: [w256 w258] -> w253
                      frame True {
                        w256 = u32 0  # Time to hold source OFF (microseconds)
                        w257 = u32 1  # Time to hold source ON (microseconds)
                      }
                      frame False {
                        w258 = u32 1  # Time to hold source OFF (microseconds)
                        w259 = u32 0  # Time to hold source ON (microseconds)
                      }
                    }
                    n188 = call "Arduino_Timed_Release.vi"("Time to hold source ON (microseconds)"=w254, "Time to hold source OFF (microseconds)"=w253, "Number of cycles"=u16 1) -> ()  [unwired: 2 out]
                  }
                  frame #1 {
                    n189 = Greater Than 0?(x=w260) -> (x > 0?=w261:bool)
                    n190 = case shown="True" w261 {
                      tunnel: w260 -> [_ w262]
                      frame False {
                      }
                      frame True {
                        n191 = call "Wait_Seconds_with_display.vi"("Message"="Est Source", "Seconds to wait"=w262) -> ()  [unwired: 2 out]
                      }
                    }
                  }
                }
              }
              frame True {
                n192 = global read "Gas_management_global.vi" "Source Live Last changed"() -> (w268:timestamp)
                n193 = Get Date/Time In Seconds() -> (seconds since 1Jan1904=w269:timestamp)
                n194 = Subtract(x=w269, y=w268) -> (x-y=w267:dbl)
                n195 = Subtract(x=w264, y=w267) -> (x-y=w265:dbl)
                n196 = call "Wait_Seconds_with_display.vi"("Message"="Est Source", "Seconds to wait"=w265) -> ()  [unwired: 2 out]
              }
            }
          }
        }
      }
      frame #9 {
        # "Moved flusher from 23 to 28- after file is written!"
        # "This allows ad-hoc locally-added comments as well as MR-injected ones.\nMaybe we shouldn't allow local in MR tho...\n\nTCRL 20240602"
        # "Assemble Comments"
        n197 = local read "Comments"() -> (w273:string)
        n198 = Concatenate Strings(w270, w273) -> (w272:string)
        n199 = call "Text_without_format.vi"("Input string"=w272) -> ("Output string"=w271:string)
        n200 = local write "Comments"(w271) -> ()
        n201 = global write "Meas_global.vi" "Comments"(w271) -> ()
      }
      frame #10 {
        # "Saving data or not..?"
        n202 = global read "Trav_pos_global.vi" "Meas Setup Number"() -> (w280:i32)
        n203 = global read "Meas_global.vi" "Post Process"() -> (w287:T2)
        n204 = global read "Meas_global.vi" "Remote control"() -> (w296:bool)
        n205 = call "Current_Filepath.vi"("Short_Name"="Res" ("Data Type"), "Filename in"="Results file", "Data Type"="Results") -> ("Filename Out"=w279:path)  [unwired: 1 in, 1 out]
        n206 = Equal?(x=w287, y=Post_Process."Take New Data" ("Post Process")) -> (x = y?=w286:bool)
        n207 = case shown="1, Default" w280 {
          selector: w280 -> [_ w304]
          tunnel: [w303 w306] -> w281
          tunnel: w279 -> [w303 w313]
          frame 0 {
          }
          frame 1, Default {
            n208 = Add(x=96, y=w304) -> (x+y=w315:i32)
            n209 = Build Array(w315) -> (w316:i32[])
            n210 = Strip Path(path=w313) -> (stripped path=w307:path, name=w312:string)
            n211 = Byte Array To String(unsigned byte array=w316) -> (string=w310:string)
            n212 = call "Add_filename_suffix.vi"("Filename"=w312) -> ("Original Suffix"=w309:string, "Base name"=w311:string)  [unwired: 1 in, 2 out]
            n213 = Format Into String(format string="%s_%s%s", w311, w310, w309) -> (resulting string=w308:string)  [unwired: 2 in, 1 out]
            n214 = Build Path(base path=w307, name or relative path=w308) -> (appended path=w306:path)
          }
        }
        n215 = Not Equal?(x=Setup."Run Program" ("setup"), y=w299) -> (x != y?=w285:bool)
        n216 = Equal?(x="File", y=Save_Data."Save No Data" ("File")) -> (x = y?=w294:bool)
        n217 = Compound Arithmetic op=AND(w294, invert w296, w286, invert w285, w275) -> (w295:bool)
        n218 = while {
          shift-left: _ -> [w321]
          shift-right: [w318] -> _
          tunnel: "File" -> [w319]
          tunnel: [w322] -> w293
          tunnel: w295 -> [w318]
          stop <- FALSE continue-if-true
          n219 = Compound Arithmetic op=AND(w318, invert w321) -> (w320:bool)
          n220 = case shown="True" w320 {
            tunnel: [w323 w326] -> w322
            tunnel: w319 -> [w323 _]
            frame False {
            }
            frame True {
              n221 = Two Button Dialog(message="Do you wish to save the data?", 1:"Save Data" ("F button name (\"Cancel\")"), 2:"Save No Data" ("T button name (\"OK\")")) -> (T button?=w327:bool)
              n222 = Select(t=Save_Data."Save No Data" ("File"), s=w327, f=Save_Data."Save Data" ("File")) -> (s? t:f=w326:T4)
            }
          }
        }
        n223 = Equal?(x=Save_Data."Save No Data" ("File"), y=w293) -> (x = y?=w283:bool)
        n224 = And(x=w296, y=w286) -> (x .and. y?=w292:bool)
        n225 = Or(x=w283, y=w285) -> (x .or. y?=w298:bool)
        n226 = case shown="True" w298 {
          tunnel: w281 -> [w342 w350]
          tunnel: [w341 w350] -> w301
          tunnel: "Raw data file" -> [w340 w351]
          tunnel: [w335 w351] -> w290
          tunnel: w299 -> [w339 _]
          tunnel: w293 -> [w338 _]
          tunnel: [w336 T15."Save no data" ("File output")] -> w288
          tunnel: [w337 w348] -> w282
          tunnel: w292 -> [_ w345]
          tunnel: w285 -> [_ w344]
          tunnel: w275 -> [w334 _]
          frame False {
            n227 = call "File_setup.vi"("Measurement is top level?"=w334, "Results file"=w342, "Raw data file"=w340, "setup"=w339, "File"=w338) -> ("Results file output"=w341:path, "Raw data file output"=w335:path, "Raw data option"=w337:enum16{"Save raw data", "Raw data not saved"}, "File output"=w336:T15)
          }
          frame True {
            n228 = global read "Meas_global.vi" "Raw data option"() -> (w347:enum16{"Save raw data", "Raw data not saved"})
            n229 = Compound Arithmetic op=AND(w345, invert w344) -> (w343:bool)
            n230 = Select(t=w347, s=w343, f=enum16{"Save raw data", "Raw data not saved"}."Raw data not saved" ("Raw data option")) -> (s? t:f=w348:enum16{"Save raw data", "Raw data not saved"})
          }
        }
        n231 = case shown="\"Save raw data\"" w282 {
          tunnel: w290 -> [w331 w333]
          tunnel: [w331 w332] -> w289
          frame "Raw data not saved" {
          }
          frame "Save raw data" {
            n232 = call "Find_Unique_Filename.vi"("Path In"=w333) -> ("Unique Path Out"=w332:path)  [unwired: 1 in, 1 out]
          }
        }
        n233 = global write "Meas_global.vi" "File"(w288) -> ()
        n234 = global write "Meas_global.vi" "Results file"(w301) -> ()
        n235 = local write "Results file"(w301) -> ()
        n236 = global write "Meas_global.vi" "Raw data option"(w282) -> ()
        n237 = local write "File"(w293) -> ()
        n238 = global write "Meas_global.vi" "Raw data file"(w289) -> ()
        n239 = local write "Raw data file"(w289) -> ()
      }
      frame #11 {
        # "Populate Plot strings"
        n240 = local read "Block average display control"() -> (w355:cluster{"Name":string, "Include":bool}[])
        n241 = global read "Meas_global.vi" "Analysis Info cluster"() -> (w352:T23[])
        n242 = for {
          tunnel: w352 -> [w363] mode=indexing
          tunnel: w355 -> [w362]
          tunnel: [w358] -> w354 mode=indexing
          tunnel: [w359] -> w353 mode=indexing
          i -> [w361]
          n243 = Index Array(array=w362, index=w361) -> (element=w360:cluster{"Name":string, "Include":bool})
          n244 = Unbundle By Name(w363) -> ("Label"=w358:string)
          n245 = Bundle By Name(cluster=w360, "Name"=w358) -> (w359:cluster{"Name":string, "Include":bool})
        }
        n246 = local write "Block average display control"(w353) -> ()
        n247 = Build Array (concatenate)("Nothing", w354) -> (w356:string[])
        n248 = property on="Plot 1" class="Ring (strict)"("Strings []"=w356) -> ()  [unwired: 2 in, 2 out]
        n249 = property on="Plot 1" class="Ring (strict)"("Strings []"=w356) -> ()  [unwired: 2 in, 2 out]
        n250 = property on="Plot 2" class="Ring (strict)"("Strings []"=w356) -> ()  [unwired: 2 in, 2 out]
        n251 = property on="Plot 2" class="Ring (strict)"("Strings []"=w356) -> ()  [unwired: 2 in, 2 out]
      }
      frame #12 {
        n252 = global read "Meas_global.vi" "Analysis Info cluster"() -> (w364:T23[])
        n253 = stacked-sequence {
          seq-local: [_ _ w444 _ _ _] -> [_ _ _ w455 _ _]
          seq-local: [_ w410 _ _ _ _] -> [_ _ w445 _ _ _]
          seq-local: [_ w412 _ _ _ _] -> [_ _ w443 _ _ _]
          seq-local: [w367 _ _ _ _ _] -> [_ w409 _ _ _ _]
          tunnel: w364 -> [w369 w418 w447 _ w490 w494]
          frame #0 {
            n254 = for {
              tunnel: w369 -> [w397] mode=indexing
              tunnel: [w394] -> w366 mode=indexing if=w393
              i -> [w395]
              n255 = Unbundle By Name(w397) -> ("Inst type"=w396:T12, "Device"=w392:string)
              n256 = case shown="\"Cross wire 1\"" w396 {
                tunnel: w395 -> [_ w405]
                tunnel: [i32[] [] w404] -> w394
                tunnel: [FALSE w400] -> w393
                tunnel: w392 -> [_ w402]
                frame "Raw voltage", Default {
                }
                frame "Cross wire 1" {
                  n257 = Increment(x=w405) -> (x+1=w406:i32)
                  n258 = Match Pattern(string=w402, regular expression="Derived") -> (offset past match=w401:i32)  [unwired: 1 in, 3 out]
                  n259 = Less Than 0?(x=w401) -> (x < 0?=w400:bool)
                  n260 = Build Array(w405, w406) -> (w404:i32[])
                }
              }
            }
            n261 = for {
              tunnel: w369 -> [w389] mode=indexing
              tunnel: [w388] -> w365 mode=indexing if=w387
              i -> [w388]
              n262 = Unbundle By Name(w389) -> ("Inst type"=w390:T12)
              n263 = Equal?(x=w390, y=Inst_type."LDA Vel" ("Inst type")) -> (x = y?=w387:bool)
            }
            n264 = Array Size(array=w365) -> (size(s)=w368:i32)
            n265 = case shown="2" w368 {
              tunnel: [w370 w371 w372 w383] -> w367
              tunnel: w366 -> [w370 w371 w373 w384]
              tunnel: w365 -> [_ _ w377 w386]
              frame 0 {
              }
              frame 1 {
              }
              frame 2 {
                n266 = Index Array(array=w377) -> (element #1=w376:i32, element #2=w375:i32)  [unwired: 2 in]
                n267 = Build Array(w376, w375) -> (w374:i32[])
                n268 = Build Array (concatenate)(w373, w374) -> (w372:i32[][])
              }
              frame 3, Default {
                n269 = Index Array(array=w386) -> (element #1=w382:i32, element #2=w381:i32, element #3=w380:i32)  [unwired: 3 in]
                n270 = Build Array(w382, w381) -> (w385:i32[])
                n271 = Build Array(w382, w380) -> (w379:i32[])
                n272 = Build Array(w381, w380) -> (w378:i32[])
                n273 = Build Array (concatenate)(w384, w385, w379, w378) -> (w383:i32[][])
              }
            }
          }
          frame #1 {
            n274 = for {
              tunnel: w418 -> [w440] mode=indexing
              tunnel: [w439] -> w422
              stop <- w439 stop-if-true
              n275 = Unbundle By Name(w440) -> ("Inst type"=w441:T12)
              n276 = Equal?(x=w441, y=Inst_type."LDA Vel" ("Inst type")) -> (x = y?=w439:bool)
            }
            n277 = global read "Meas_global.vi" "Pre Setup String"() -> (w417:string)
            n278 = call "Correlation_Setup.vi"("Input string"=w417) -> ("Correlate"=w408:i32[][], "Error?"=w416:bool)
            n279 = global read "Meas_global.vi" "Post Process"() -> (w419:T2)
            n280 = for {
              tunnel: w409 -> [w425] mode=indexing
              tunnel: w408 -> [w426]
              tunnel: [w425] -> w407 mode=indexing if=w423
              n281 = for {
                tunnel: w425 -> [w429]
                tunnel: w426 -> [w428] mode=indexing
                tunnel: [w427] -> w424
                stop <- w427 stop-if-true
                n282 = Equal?(x=w428, y=w429) -> (x = y?=w427:bool)
              }
              n283 = Not(x=w424) -> (.not. x?=w423:bool)
            }
            n284 = Equal?(x=w419, y=Post_Process."Post Process Raw Data File" ("Post Process")) -> (x = y?=w421:bool)
            n285 = Build Array (concatenate)(w408, w407) -> (w410:i32[][])
            n286 = Compound Arithmetic op=AND(w422, w421, w416) -> (w414:bool)
            n287 = case shown="\"Cross correlation off\"" "Correlate?" {
              tunnel: w410 -> [w434 _ _]
              tunnel: [w432 FALSE FALSE] -> w415
              frame "Cross correlation off" {
                n288 = Array Size(array=w434) -> (size(s)=w436:i32[])
                n289 = Index Array(array=w436, index=0) -> (element=w433:i32)
                n290 = Greater Than 0?(x=w433) -> (x > 0?=w432:bool)
              }
              frame "Show correlation panel" {
              }
              frame "Correlate without activating panel" {
              }
            }
            n291 = Or(x=w415, y=w414) -> (x .or. y?=w413:bool)
            n292 = case shown="True" w413 {
              tunnel: [w430 w431] -> w412
              tunnel: "Correlate?" -> [w430 _]
              frame False {
              }
              frame True {
                w431 = T8."Correlate without activating panel" ("Correlate?")
                n293 = local write "Correlate?"(w431) -> ()
              }
            }
          }
          frame #2 {
            n294 = for {
              tunnel: w447 -> [w454] mode=indexing
              tunnel: [w453] -> w446 mode=indexing
              n295 = Unbundle By Name(w454) -> ("Inst name"=w453:string)
            }
            n296 = case shown="\"Show correlation panel\"" w443 {
              tunnel: w446 -> [_ _ w452]
              tunnel: w445 -> [_ w449 w451]
              tunnel: [i32[][] [] ("Correlate Out") w449 w450] -> w444
              frame "Cross correlation off" {
              }
              frame "Correlate without activating panel" {
              }
              frame "Show correlation panel" {
                n297 = call "Select Correlation pairs.vi"("Correlate In"=w451, "Instrument names"=w452) -> ("Correlate Out"=w450:i32[][])  [unwired: 1 in]
              }
            }
          }
          frame #3 {
            n298 = for {
              tunnel: w455 -> [w466] mode=indexing
              shift-right: [w469] -> _
              shift-left: string[] [] -> [w470]
              tunnel: [w466] -> w457 mode=indexing if=w468
              n299 = Index Array(array=w466) -> (element #1=w465:i32, element #2=w463:i32)  [unwired: 2 in]
              n300 = Not Equal?(x=w465, y=w463) -> (x != y?=w464:bool)
              n301 = Format Into String(format string="%d and %d;", w465, w463) -> (resulting string=w467:string)  [unwired: 2 in, 1 out]
              n302 = Search 1D Array(1D array=w470, element=w467) -> (index of element=w471:i32)  [unwired: 1 out]
              n303 = case shown="-1" w471 {
                tunnel: w467 -> [_ w482]
                tunnel: w470 -> [w474 w481]
                tunnel: [w474 w480] -> w469
                tunnel: [FALSE w475] -> w468
                tunnel: w466 -> [_ w479]
                tunnel: w464 -> [_ w476]
                frame Default {
                }
                frame -1 {
                  n304 = Greater Or Equal To 0?(x=w479) -> (x >= 0?=w478:bool[])
                  n305 = Build Array (concatenate)(w481, w482) -> (w480:string[])
                  n306 = And Array Elements(Boolean array=w478) -> (logical AND=w477:bool)
                  n307 = And(x=w477, y=w476) -> (x .and. y?=w475:bool)
                }
              }
            }
            n308 = Array Size(array=w457) -> (size(s)=w462:i32[])
            n309 = global write "Meas_global.vi" "correlate"(w457) -> ()
            n310 = Index Array(array=w462, index=0) -> (element=w459:i32)
            n311 = Equal To 0?(x=w459) -> (x = 0?=w460:bool)
            n312 = case shown="False" w460 {
              tunnel: [T8."Correlate without activating panel" ("Correlate?") T8."Cross correlation off" ("Correlate?")] -> w458
              frame False {
              }
              frame True {
              }
            }
            n313 = local write "Correlate?"(w458) -> ()
          }
          frame #4 {
            n314 = Array Size(array=w490) -> (size(s)=w486:i32)
            n315 = Initialize Array(T16 {"Weighting"=[], "Voltage"=[], "Eng Values"=[]} ("Time Trace"), w486) -> (w489:T16[])
            n316 = Initialize Array(-1, w486) -> (w485:i32[])
            n317 = global write "Meas_global.vi" "Time Trace"(w489) -> ()
            n318 = global write "Meas_global.vi" "Time Array Index"(w485) -> ()
          }
          frame #5 {
            n319 = global read "Meas_global.vi" "Duplicate channels"() -> (w491:i32[])
            n320 = case shown="False" "Select Duplicate Channels" {
              tunnel: w494 -> [w497 w518]
              tunnel: w491 -> [w496 w520]
              tunnel: [w496 w519] -> w492
              frame False {
                n321 = for {
                  tunnel: w497 -> [w515]
                  tunnel: w496 -> [w514] mode=indexing
                  tunnel: [w512] -> w500 mode=indexing
                  n322 = Index Array(array=w515, index=w514) -> (element=w513:T23)
                  n323 = Unbundle By Name(w513) -> ("Stats"=w512:enum16{"None", "Basic", "Full"})
                }
                n324 = Array Max & Min(array=w500) -> (max value=w495:enum16{"None", "Basic", "Full"}, min value=w499:enum16{"None", "Basic", "Full"})  [unwired: 2 out]
                n325 = Greater?(x=w495, y=w499) -> (0:w498:bool)
                n326 = case shown="True" w498 {
                  tunnel: w497 -> [_ w503]
                  tunnel: w496 -> [_ w504]
                  tunnel: w495 -> [_ w502]
                  frame False {
                  }
                  frame True {
                    n327 = for {
                      tunnel: w504 -> [w508] mode=indexing
                      shift-right: [w506] -> w501
                      shift-left: w503 -> [w507]
                      tunnel: w502 -> [w505]
                      n328 = in-place {
                        in-place-border: w505 -> [w509]
                        n329 = in-place-array #1(w507, w508) -> (w511:T23)
                        n330 = Bundle By Name(cluster=w511, "Stats"=w509) -> (w510:T23)
                        n331 = in-place-array #1(w510) -> (w506:T23[])  [unwired: 1 out]
                      }
                    }
                    n332 = global write "Meas_global.vi" "Analysis Info cluster"(w501) -> ()
                  }
                }
              }
              frame True {
                n333 = for {
                  tunnel: w518 -> [w527] mode=indexing
                  tunnel: [w526] -> w516 mode=indexing
                  n334 = Unbundle By Name(w527) -> ("Inst name"=w526:string)
                }
                n335 = for {
                  shift-right: [w529] -> w523
                  shift-left: string[] [] -> [w530]
                  tunnel: w520 -> [w532]
                  tunnel: [w528] -> w522 mode=indexing
                  tunnel: w516 -> [w528] mode=indexing
                  i -> [w533]
                  n336 = Search 1D Array(1D array=w532, element=w533) -> (index of element=w531:i32)  [unwired: 1 out]
                  n337 = case shown="0, Default" w531 {
                    tunnel: w530 -> [w536 w537]
                    tunnel: w528 -> [w535 _]
                    tunnel: [w534 w537] -> w529
                    frame 0, Default {
                      n338 = Build Array (concatenate)(w536, w535) -> (w534:string[])
                    }
                    frame -1 {
                    }
                  }
                }
                n339 = local write "Select Duplicate Channels"(FALSE ("Select Local ADAM Channels")) -> ()
                n340 = call "Select_Strings.vi"("Available Ch names"=w522, "Message"="Please select similar instruments whose results columns will be combined", "Selector mode"=T17."Zero or more", "Desired Ch names (in)"=w523) -> ("Ch Indicies Chosen"=w519:i32[])  [unwired: 1 in, 3 out]
              }
            }
            n341 = global write "Meas_global.vi" "Duplicate channels"(w492) -> ()
          }
        }
      }
      frame #13 {
        n342 = stacked-sequence {
          seq-local: [w548 _] -> [_ w570]
          tunnel: w539 -> [w547 _]
          tunnel: w538 -> [w541 _]
          frame #0 {
            n343 = Equal?(x=w541, y=Setup."Run Program" ("setup")) -> (x = y?=w540:bool)
            n344 = call "LDA+_An_Analysis_mode.vi"("Second Graph"="Second Graph", "Running Code?"=w540, "First Graph"="First Graph") -> ("Second Graph out"=w543:T7, "First Graph out"=w545:T7)  [unwired: 5 out]
            n345 = case shown="False" w547 {
              tunnel: [w558 w569] -> w546
              tunnel: w545 -> [w557 w569]
              tunnel: [w556 w568] -> w544
              tunnel: w543 -> [w555 w568]
              frame False {
                w553 = Graph_Type."Show no graph" ("Plot Type")
                n346 = Unbundle By Name(w557) -> ("Save graph"=w559:u16)
                n347 = Unbundle By Name(w555) -> ("Save graph"=w554:u16)
                n348 = case shown="0, Default" w559 {
                  tunnel: [w565 w567] -> w558
                  tunnel: w557 -> [w566 w567]
                  tunnel: w553 -> [w564 _]
                  frame 0, Default {
                    n349 = Bundle By Name(cluster=w566, "Plot Type"=w564) -> (w565:T7)
                  }
                  frame 1 {
                  }
                }
                n350 = case shown="0, Default" w554 {
                  tunnel: [w561 w563] -> w556
                  tunnel: w555 -> [w562 w563]
                  tunnel: w553 -> [w560 _]
                  frame 0, Default {
                    n351 = Bundle By Name(cluster=w562, "Plot Type"=w560) -> (w561:T7)
                  }
                  frame 1 {
                  }
                }
              }
              frame True {
              }
            }
            n352 = local write "Second Graph"(w544) -> ()
            n353 = local write "First Graph"(w546) -> ()
            n354 = global write "Meas_global.vi" "Second Graph"(w544) -> ()
            n355 = global write "Meas_global.vi" "First Graph"(w546) -> ()
            n356 = Unbundle By Name(w544) -> ("Plot Type"=w552:T6)
            n357 = Unbundle By Name(w546) -> ("Plot Type"=w551:T6)
            n358 = Build Array(w551, w552) -> (w548:T6[])
          }
          frame #1 {
            n359 = global read "Meas_global.vi" "Insts for plotting"() -> (w571:u16[][])
            n360 = for {
              tunnel: w571 -> [w573] mode=indexing
              tunnel: w570 -> [w572] mode=indexing
              i -> [w574]
              n361 = stacked-sequence {
                seq-local: [w577 _] -> [_ w595]
                seq-local: [w578 _] -> [_ w594]
                tunnel: w574 -> [_ w596]
                tunnel: w573 -> [w575 _]
                tunnel: w572 -> [_ w593]
                frame #0 {
                  n362 = property on="Plot 1" class="Ring (strict)"() -> ("Strings []"=w576:string[])  [unwired: 2 in, 2 out]
                  n363 = Array To Cluster(array=w575) -> (cluster=w581:T25)
                  n364 = Unbundle(w581) -> ("Insts for plotting[0]"=w580:u16, "Insts for plotting[1]"=w579:u16)
                  n365 = Index Array(array=w576, index=w580) -> (element=w577:string)
                  n366 = Index Array(array=w576, index=w579) -> (element=w578:string)
                }
                frame #1 {
                  n367 = case shown="\"Spectrum\"" w593 {
                    tunnel: [u8 0 u8 0 u8 0 u8 0 u8 0 u8 1 u8 0] -> w592
                    tunnel: [u8 0 u8 0 u8 0 u8 0 u8 1 u8 1 u8 0] -> w591
                    tunnel: [u8 0 u8 0 u8 0 u8 0 u8 1 u8 1 u8 0] -> w590
                    tunnel: [u8 0 u8 0 u8 0 u8 0 u8 1 u8 0 u8 0] -> w589
                    tunnel: [FALSE TRUE TRUE TRUE TRUE TRUE TRUE] -> w586
                    tunnel: [u8 0 u8 1 u8 1 u8 2 u8 2 u8 0 u8 2] -> w585
                    tunnel: [u8 0 u8 4 u8 1 u8 2 u8 1 u8 0 u8 1] -> w584
                    tunnel: ["" "Time (s)" "Time (s)" "" "" "" ""] -> w583
                    tunnel: ["" "Voltage" "Velocity" "" "" "" ""] -> w582
                    frame "Show no graph" {
                    }
                    frame "Voltage trace" {
                    }
                    frame "Velocity trace" {
                    }
                    frame "Vel histogram" {
                    }
                    frame "Spectrum" {
                    }
                    frame "f.E(f) v Log f" {
                    }
                    frame "Auto-Corr" {
                    }
                  }
                  n368 = case shown="1" w596 {
                    tunnel: w586 -> [w609 w622]
                    tunnel: w592 -> [w608 w621]
                    tunnel: w591 -> [w607 w620]
                    tunnel: w590 -> [w606 w619]
                    tunnel: w589 -> [w605 w618]
                    tunnel: u32 0 -> [w604 w617]
                    tunnel: u32 1 -> [w603 w615]
                    tunnel: w595 -> [w602 w616]
                    tunnel: w594 -> [w601 w614]
                    tunnel: w585 -> [w600 w613]
                    tunnel: w584 -> [w599 w612]
                    tunnel: w583 -> [w598 w611]
                    tunnel: w582 -> [w597 w610]
                    frame 0, Default {
                      n369 = property on="First plot" class="XYGraph (strict)"("Visible"=w609, "X Scale.Format & Precision:Format"=w608, "X Scale.Mapping Mode"=w607, "Y Scale.Format & Precision:Format"=w606, "Y Scale.Mapping Mode"=w605, "Active Plot"=w604, "Plot.Plot Name"=w602, "Active Plot"=w603, "Plot.Plot Name"=w601, "X Scale.Format & Precision:Precision"=w600, "Y Scale.Format & Precision:Precision"=w599, "XScale.NameLbl.Text"=w598, "YScale.NameLbl.Text"=w597) -> ()  [unwired: 2 in, 2 out]
                    }
                    frame 1 {
                      n370 = property on="2nd plot" class="XYGraph (strict)"("Visible"=w622, "X Scale.Format & Precision:Format"=w621, "X Scale.Mapping Mode"=w620, "Y Scale.Format & Precision:Format"=w619, "Y Scale.Mapping Mode"=w618, "Active Plot"=w617, "Plot.Plot Name"=w616, "Active Plot"=w615, "Plot.Plot Name"=w614, "X Scale.Format & Precision:Precision"=w613, "Y Scale.Format & Precision:Precision"=w612, "XScale.NameLbl.Text"=w611, "YScale.NameLbl.Text"=w610) -> ()  [unwired: 2 in, 2 out]
                    }
                  }
                }
              }
            }
          }
        }
      }
      frame #14 {
        n371 = local read "Second Graph"() -> (w697:T7)
        n372 = local read "First Graph"() -> (w696:T7)
        n373 = Unbundle By Name(w696) -> ("Plot 1"=w689:u16, "Plot 2"=w690:u16)
        n374 = Unbundle By Name(w697) -> ("Plot 1"=w691:u16, "Plot 2"=w692:u16)
        n375 = Build Array(w689, w690) -> (w693:u16[])
        n376 = Build Array(w691, w692) -> (w694:u16[])
        n377 = global read "Meas_global.vi" "Analysis Info cluster"() -> (w698:T23[])
        n378 = Decrement(x=w693) -> (x-1=w687:u16[])
        n379 = Decrement(x=w694) -> (x-1=w695:u16[])
        n380 = for {
          tunnel: w698 -> [w706]
          tunnel: w687 -> [w705] mode=indexing
          shift-right: [w699] -> _
          shift-left: u32 0 -> [w701]
          i -> [w700]
          n381 = Index Array(array=w706, index=w705) -> (element=w707:T23)
          n382 = Unbundle By Name(w707) -> ("Colour"=w702:u32)
          n383 = Equal?(x=w702, y=w701) -> (x = y?=w704:bool)
          n384 = Select(t=u32 13434624, s=w704, f=w702) -> (s? t:f=w699:u32)
          n385 = property on="First plot" class="XYGraph (strict)"("Active Plot"=w700, "Plot.Plot Color"=w699, "Plot.Fill/Point Color"=w699) -> ()  [unwired: 2 in, 2 out]
        }
        n386 = for {
          tunnel: w698 -> [w715]
          tunnel: w695 -> [w714] mode=indexing
          shift-right: [w710] -> _
          shift-left: u32 0 -> [w708]
          i -> [w713]
          n387 = Index Array(array=w715, index=w714) -> (element=w716:T23)
          n388 = Unbundle By Name(w716) -> ("Colour"=w709:u32)
          n389 = Equal?(x=w709, y=w708) -> (x = y?=w712:bool)
          n390 = Select(t=u32 13434624, s=w712, f=w709) -> (s? t:f=w710:u32)
          n391 = property on="2nd plot" class="XYGraph (strict)"("Active Plot"=w713, "Plot.Plot Color"=w710, "Plot.Fill/Point Color"=w710) -> ()  [unwired: 2 in, 2 out]
        }
      }
      frame #15 {
        n392 = global read "Meas_global.vi" "Remote control"() -> (w722:bool)
        n393 = global read "Meas_global.vi" "Post Process"() -> (w725:T2)
        n394 = Equal?(x=Setup."Run Program" ("setup"), y=w721) -> (x = y?=w717:bool)
        n395 = Equal?(x=Post_Process."Take New Data" ("Post Process"), y=w725) -> (x = y?=w718:bool)
        n396 = Compound Arithmetic op=AND(invert w719, invert w722, w718, w717) -> (w723:bool)
        n397 = case shown="True" w723 {
          frame False {
          }
          frame True {
            n398 = global read "Meas_global.vi" "Extra command String"() -> (w728:string)
            n399 = global read "Meas_global.vi" "Averaging time (min)"() -> (w726:dbl)
            n400 = global read "Extra_Commands_Global.vi" "Block Length (s)"() -> (w730:string)
            n401 = call "Extra_Commands.vi"("String to Search"=w728, "Command"=w730) -> ("Numeric Value"=w727:dbl, "Command Found"=w729:bool)  [unwired: 1 in, 3 out]
            n402 = Multiply(x=w726, y=60.0) -> (x*y=w732:dbl)
            n403 = case shown="True" w729 {
              tunnel: [1 w741] -> w734
              tunnel: w732 -> [w735 w739]
              tunnel: [w735 w738] -> w731
              tunnel: w727 -> [_ w737]
              frame False {
              }
              frame True {
                n404 = Greater?(x=w737, y=w739) -> (0:w740:bool)
                n405 = case shown="False" w740 {
                  tunnel: w737 -> [w742 _]
                  tunnel: [w746 1] -> w741
                  tunnel: w739 -> [w744 w747]
                  tunnel: [w742 w747] -> w738
                  frame False {
                    n406 = Divide(x=w744, y=w742) -> (x/y=w745:dbl)
                    n407 = Round To Nearest(number=w745) -> (nearest integer value=w743:dbl)
                    n408 = To Long Integer(number=w743) -> (32bit integer=w746:i32)
                  }
                  frame True {
                  }
                }
              }
            }
            n409 = local write "Time per Block (s)"(w731) -> ()
            n410 = global write "Meas_global.vi" "Time per Block (s)"(w731) -> ()
            n411 = global write "Meas_global.vi" "Requested No of blocks"(w734) -> ()
            n412 = local write "No of Blocks"(w734) -> ()
          }
        }
      }
      frame #16 {
        n413 = case shown="\"Run Program\"" w749 {
          frame "Run Program" {
            n414 = call "Read_calibration_files.vi"() -> ()  [unwired: 1 out]
            n415 = global read "Meas_global.vi" "Post Process"() -> (w750:T2)
            n416 = case shown="\"Take New Data\"" w750 {
              frame "Take New Data" {
                n417 = global read "Meas_global.vi" "Requested No of blocks"() -> (w753:i32)
                n418 = global read "Meas_global.vi" "Time per Block (s)"() -> (w759:dbl)
                n419 = Multiply(x=w753, y=w759) -> (x*y=w760:dbl)
                n420 = Multiply(x=3, y=w753) -> (x*y=w751:i32)
                n421 = Add(x=w760, y=120.0) -> (x+y=w755:dbl)
                n422 = Add(x=w751, y=w755) -> (x+y=w754:dbl)
                n423 = call "Program_Active_Client.vi"("Mode"=enum16{"Program Active", "Traverse Level State"}."Program Active", "Time till next contact (Sec)"=w754, "Traverse level State"=Traverse_Level_State."Running") -> ()  [unwired: 3 out]
              }
              frame "Post Process Raw Data File" {
              }
            }
          }
          frame "Show Setup", Default {
          }
        }
      }
      frame #17 {
        n424 = global write "Meas_global.vi" "Setup complete?"(TRUE ("Setup complete?")) -> ()
      }
      frame #18 {
        # "*** HERE IS WHERE THE DATA GETS TAKEN ***"
        # "Taking Measurement Blocks"
        # "TAKE THE DATA IN HERE"
        n425 = case shown="\"Run Program\"" w763 {
          tunnel: w762 -> [w764 _]
          frame "Run Program" {
            n426 = while {
              tunnel: w764 -> [w765]
              i -> [w766]
              stop <- w767 stop-if-true
              n427 = Increment(x=w766) -> (x+1=w768:i32)
              n428 = stacked-sequence {
                seq-local: [_ _ _ _ _ _ "Block average display control" _ _ _] -> [_ _ _ _ _ _ _ w900 _ _]
                seq-local: [_ _ _ _ _ _ _ w898 _ _] -> [_ _ _ _ _ _ _ _ w905 _]
                seq-local: [_ w772 _ _ _ _ _ _ _ _] -> [_ _ w859 _ _ _ _ _ _ _]
                seq-local: [_ _ w855 _ _ _ _ _ _ _] -> [_ _ _ _ _ _ _ _ _ _]
                seq-local: [_ _ _ _ _ w886 _ _ _ _] -> [_ _ _ _ _ _ _ _ _ w908]
                tunnel: w768 -> [w769 w770 w858 _ _ w887 w893 _ _ _]
                tunnel: [_ _ _ _ _ _ _ _ _ w909] -> w767
                tunnel: w765 -> [_ _ _ _ w865 _ _ _ _ _]
                frame #0 {
                  n429 = global write "Meas_global.vi" "Current Block No"(w769) -> ()
                  "Current Block No" <- w769
                }
                frame #1 {
                  n430 = for {
                    N: 2 -> [_]
                    tunnel: [w776] -> w772
                    tunnel: w770 -> [w774]
                    i -> [w773]
                    stop <- w775 continue-if-true
                    n431 = stacked-sequence {
                      seq-local: [w777 _ _] -> [_ _ w817]
                      tunnel: [_ _ w822] -> w776
                      tunnel: [_ _ w820] -> w775
                      tunnel: w774 -> [_ _ w819]
                      tunnel: w773 -> [_ _ w818]
                      frame #0 {
                        w778 = sgl 0.0 ("progress")
                        w784 = string[] [] ("Plug in titles")
                        n432 = global read "Meas_global.vi" "Time Array Index"() -> (w782:i32[])
                        n433 = global write "Meas_global.vi" "Unique Times"(cluster{"Time (s)":dbl[]}[] [] ("Unique Times")) -> ()
                        n434 = local read "Time per Block (s)"() -> (w777:dbl)
                        n435 = Array Size(array=w782) -> (size(s)=w781:i32)
                        n436 = Initialize Array(-1, w781) -> (w780:i32[])
                        n437 = property on="progress" class="Slide (strict)"("Scale.Maximum"=w777, "Scale.Minimum"=w778, "Value"=w778) -> ()  [unwired: 2 in, 2 out]
                        n438 = global write "Meas_global.vi" "Time Array Index"(w780) -> ()
                        n439 = global write "Dynamic_call_global.ph.vi" "Plug in titles"(w784) -> ()
                        n440 = global write "Dynamic_call_global.ph.vi" "Plug in values"(w784) -> ()
                        n441 = local write "blockDone"(FALSE ("blockDone")) -> ()
                      }
                      frame #1 {
                        n442 = global read "Dynamic_call_global.ph.vi" "Initial Plug Ins Extra"() -> (w802:string[])
                        n443 = global read "Dynamic_call_global.ph.vi" "Initial Plug Ins"() -> (w801:string[])
                        n444 = global read "Meas_global.vi" "Acquisition_Plug_Ins to Run"() -> (w793:string[])
                        n445 = global read "Meas_global.vi" "Analysis Info cluster"() -> (w806:T23[])
                        n446 = Build Array (concatenate)(w801, w802) -> (w803:string[])
                        n447 = for {
                          tunnel: w806 -> [w816]
                          tunnel: w793 -> [w815] mode=indexing
                          shift-right: [w811] -> w807
                          shift-left: 2 -> [w812]
                          n448 = call "Device ID Ports.vi"("Analysis Info cluster"=w816, "DAQdeviceType"=w815) -> ("Device port info"=w814:T26[])  [unwired: 1 out]
                          n449 = Array Size(array=w814) -> (size(s)=w813:i32)
                          n450 = Add(x=w813, y=w812) -> (x+y=w811:i32)
                        }
                        n451 = Search 1D Array(1D array=w803, element="Initial_Plugin_Dynamixel.vi") -> (index of element=w804:i32)  [unwired: 1 in]
                        n452 = Search 1D Array(1D array=w803, element="Move_Trav_while_Meas_Blocks.vi") -> (index of element=w795:i32)  [unwired: 1 in]
                        n453 = Search 1D Array(1D array=w803, element="Source Profile Initial Plugin.vi") -> (index of element=w799:i32)  [unwired: 1 in]
                        n454 = Search 1D Array(1D array=w803, element="ESC Flight Profile Initial Plugin.vi") -> (index of element=w796:i32)  [unwired: 1 in]
                        n455 = Greater Or Equal To 0?(x=w804) -> (x >= 0?=w805:bool)
                        n456 = Greater Or Equal To 0?(x=w795) -> (x >= 0?=w798:bool)
                        n457 = Greater Or Equal To 0?(x=w796) -> (x >= 0?=w797:bool)
                        n458 = Greater Or Equal To 0?(x=w799) -> (x >= 0?=w800:bool)
                        n459 = Compound Arithmetic op=OR(w805, w798, w797, w800) -> (w792:bool)
                        n460 = case shown="True" w792 {
                          tunnel: w807 -> [w808 w810]
                          tunnel: [w808 w809] -> w791
                          frame False {
                          }
                          frame True {
                            n461 = Increment(x=w810) -> (x+1=w809:i32)
                          }
                        }
                        n462 = call <vilib>:"Create Rendezvous.vi"("size (2)"=w791) -> ("rendezvous"=w794:T27)  [unwired: 4 in, 2 out]
                        n463 = global write "Meas_global.vi" "Acquisition Rendezvous"(w794) -> ()
                      }
                      frame #2 {
                        # "*** HERE IS WHERE THE DATA GETS TAKEN ***"
                        n464 = global read "Meas_global.vi" "Post Process"() -> (w823:T2)
                        n465 = case shown="\"Take New Data\"" w823 {
                          tunnel: w817 -> [w831 _]
                          tunnel: [w830 FALSE ("stop")] -> w821
                          tunnel: w819 -> [w828 _]
                          tunnel: w818 -> [w829 _]
                          frame "Take New Data" {
                            n466 = stacked-sequence {
                              tunnel: w831 -> [_ w835 _]
                              tunnel: [_ _ w846] -> w830
                              frame #0 {
                                n467 = global read "Meas_global.vi" "Acquisition Rendezvous"() -> (w832:T27)
                                n468 = call <vilib>:"Wait at Rendezvous.vi"("ms timeout (-1)"=60000, "rendezvous"=w832) -> ()  [unwired: 3 in, 3 out]
                              }
                              frame #1 {
                                n469 = call <vilib>:"High Resolution Relative Seconds.vi"() -> ("relative seconds"=w834:dbl)
                                n470 = while {
                                tunnel: w834 -> [w844]
                                tunnel: w835 -> [w842]
                                stop <- w840 stop-if-true
                                n471 = call <vilib>:"High Resolution Relative Seconds.vi"() -> ("relative seconds"=w845:dbl)
                                n472 = Wait (ms)(milliseconds to wait=u32 100) -> ()  [unwired: 1 out]
                                n473 = local read "blockDone"() -> (w839:bool)
                                n474 = Subtract(x=w845, y=w844) -> (x-y=w837:dbl)
                                "progress" <- w837
                                n475 = Greater Or Equal?(x=w837, y=w842) -> (x >= y?=w841:bool)
                                n476 = local read "stop"() -> (w836:bool)
                                n477 = Less Than 0?(x=w837) -> (x < 0?=w838:bool)
                                n478 = Compound Arithmetic op=OR(w838, w841, w836, w839) -> (w840:bool)
                                }
                              }
                              frame #2 {
                                n479 = global read "Meas_global.vi" "stop"() -> (w847:bool)
                                n480 = local read "stop"() -> (w848:bool)
                                n481 = Or(x=w848, y=w847) -> (x .or. y?=w846:bool)
                              }
                            }
                            n482 = Equal To 0?(x=w829) -> (x = 0?=w825:bool)
                            n483 = Equal?(x=1, y=w828) -> (x = y?=w826:bool)
                            n484 = And(x=w825, y=w826) -> (x .and. y?=w824:bool)
                            n485 = case shown="True" w824 {
                              frame False {
                              }
                              frame True {
                                n486 = call "Log_Pictures.vi"() -> ()  [unwired: 12 in]
                              }
                            }
                          }
                          frame "Post Process Raw Data File" {
                          }
                        }
                        n487 = flat-sequence {
                          tunnel: [w850] -> w822
                          frame #0 {
                            n488 = call "Get_data.vi"() -> ("EOF? and Error status"=w850:bool, "Block Header"=w851:string)  [unwired: 10 out]
                            n489 = global write "Plug_in_data_global.vi" "Block Header"(w851) -> ()
                          }
                          frame #1 {
                            "blockDone" <- TRUE
                          }
                        }
                        n490 = Compound Arithmetic op=AND(w822, invert w821) -> (w820:bool)
                      }
                    }
                  }
                }
                frame #2 {
                  n491 = global write "Meas_global.vi" "Requested No of blocks"("No of Blocks") -> ()
                  n492 = property on="No of Blocks" class="DigNum (strict)"() -> ("ControlIndex"=w856:i32)  [unwired: 2 in, 2 out]
                  n493 = global read "Meas_global.vi" "stop"() -> (w853:bool)
                  n494 = Less Or Equal?(x="No of Blocks", y=w858) -> (x <= y?=w860:bool)
                  n495 = global write "Meas_global.vi" "Nblocks Index"(w856) -> ()
                  n496 = Compound Arithmetic op=OR("stop", w853, w859, w860) -> (w855:bool)
                  n497 = case shown="True" w855 {
                    tunnel: w858 -> [_ w861]
                    frame False {
                    }
                    frame True {
                      n498 = global write "Meas_global.vi" "Requested No of blocks"(w861) -> ()
                      n499 = local write "No of Blocks"(w861) -> ()
                    }
                  }
                  n500 = global write "Meas_global.vi" "Processing last block?"(w855) -> ()
                  n501 = global write "PWAtasksGLOBAL.vi" "STOP"(w855) -> ()
                }
                frame #3 {
                  n502 = call "Text_without_format.vi"("Input string"="Comments") -> ("Output string"=w862:string)
                  n503 = global write "Meas_global.vi" "Comments"(w862) -> ()
                  n504 = local write "Comments"(w862) -> ()
                }
                frame #4 {
                  n505 = global read "Meas_global.vi" "Don't Process"() -> (w864:bool)
                  n506 = case shown="True" w864 {
                    tunnel: w865 -> [w882 _]
                    frame False {
                      w869 = 0 ("index (row)")
                      w872 = 1 ("length")
                      n507 = call "Process_data.vi"("No of estimates output"="No of estimates output for when saving plots", "Measurement top level?"=w882) -> ("Vel stat display"=w876:string[][], "First Plot data Cluster"=→"First plot":cluster{"X array":dbl[], "Y array":dbl[]}[], "Second Plot Data Cluster"=→"2nd plot":cluster{"X array":dbl[], "Y array":dbl[]}[])  [unwired: 4 in, 1 out]
                      n508 = Delete From Array(array=w876, length=w872, index (row)=w869) -> (deleted portion=w875:string[][], array with subset deleted=w874:string[][])  [unwired: 1 in]
                      n509 = Array Size(array=w876) -> (size(s)=w880:i32[])
                      n510 = Delete From Array(array=w874, length=w872, index (col)=w869) -> (deleted portion=w871:string[][], array with subset deleted=→"Statistics":string[][])  [unwired: 1 in]
                      n511 = Index Array(array=w880) -> (element=w879:i32)  [unwired: 1 in]
                      n512 = Less?(x=w879, y=16) -> (x < y?=w877:bool)
                      n513 = Index Array(array=w875) -> (element=w868:string[])  [unwired: 2 in]
                      n514 = Index Array(array=w871, index (col)=w869) -> (element=w870:string[])  [unwired: 1 in]
                      n515 = case shown="True" w877 {
                        frame False {
                        }
                        frame True {
                          n516 = property on="Statistics" class="Tbl (strict)"("Index Values"=T19 {"Row"=0, "Column"=0} ("Selection Start")) -> ()  [unwired: 2 in, 2 out]
                        }
                      }
                      n517 = Split 1D Array(array=w868, index=1) -> (second subarray=w867:string[])  [unwired: 1 out]
                      n518 = property on="Statistics" class="Tbl (strict)"("Column Headers[]"=w867, "Row Headers[]"=w870) -> ()  [unwired: 2 in, 2 out]
                    }
                    frame True {
                    }
                  }
                }
                frame #5 {
                  n519 = global read "Meas_global.vi" "Processing last block?"() -> (w886:bool)
                  n520 = case shown="True" w886 {
                    tunnel: w887 -> [_ w888]
                    frame False {
                    }
                    frame True {
                      n521 = global write "Meas_global.vi" "Requested No of blocks"(w888) -> ()
                      n522 = local write "No of Blocks"(w888) -> ()
                    }
                  }
                }
                frame #6 {
                  n523 = global read "Meas_global.vi" "Actual Measurement time (min)"() -> (→"Measurement time (min)":dbl)
                  n524 = call "Display_blocks.vi"("Block No"=w893, "Block average display"="Block average display control") -> ("u^4"=→"u^4":dbl[][], "u^3"=→"u^3":dbl[][], "uv"=→"uv":dbl[][], "u^2"=→"u^2" →"Array u^2":dbl[][], "U"=→"U" →"Array U":dbl[][])  [unwired: 4 out]
                }
                frame #7 {
                  n525 = global read "Meas_global.vi" "Analysis Info cluster"() -> (w899:T23[])
                  n526 = global read "Meas_global.vi" "Diagnostic info"() -> (→"Diagnostic info":string[][])
                  n527 = for {
                    tunnel: w900 -> [w904] mode=indexing
                    tunnel: w899 -> [w901] mode=indexing
                    tunnel: [w903] -> w898 mode=indexing if=w902
                    n528 = Unbundle By Name(w904) -> ("Include"=w902:bool)
                    n529 = Unbundle By Name(w901) -> ("Colour"=w903:u32)
                  }
                }
                frame #8 {
                  n530 = for {
                    tunnel: w905 -> [w906] mode=indexing
                    i -> [w907]
                    n531 = property on="U" class="WFGraph (strict)"("Active Plot"=w907, "Plot.Plot Color"=w906, "Plot.Fill/Point Color"=w906) -> ()  [unwired: 2 in, 2 out]
                    n532 = property on="u^3" class="WFGraph (strict)"("Active Plot"=w907, "Plot.Plot Color"=w906, "Plot.Fill/Point Color"=w906) -> ()  [unwired: 2 in, 2 out]
                    n533 = property on="u^4" class="WFGraph (strict)"("Active Plot"=w907, "Plot.Plot Color"=w906, "Plot.Fill/Point Color"=w906) -> ()  [unwired: 2 in, 2 out]
                    n534 = property on="u^2" class="WFGraph (strict)"("Active Plot"=w907, "Plot.Plot Color"=w906, "Plot.Fill/Point Color"=w906) -> ()  [unwired: 2 in, 2 out]
                  }
                }
                frame #9 {
                  n535 = case shown="True" "Pause" {
                    tunnel: [w911 w913] -> w909
                    tunnel: w908 -> [w911 w912]
                    frame False {
                    }
                    frame True {
                      n536 = global read "Meas_global.vi" "Post Process"() -> (w914:T2)
                      n537 = case shown="\"Post Process Raw Data File\"" w914 {
                        tunnel: [w915 w931] -> w913
                        tunnel: w912 -> [w915 w932]
                        frame "Take New Data" {
                          n538 = call "Program_Active_Client.vi"("Mode"=enum16{"Program Active", "Traverse Level State"}."Program Active", "Time till next contact (Sec)"=12000.0, "Traverse level State"=Traverse_Level_State."Running") -> ()  [unwired: 3 out]
                          n539 = while {
                            i -> [w922]
                            stop <- w923 continue-if-true
                            n540 = Quotient & Remainder(x=w922, y=10) -> (x-y*floor(x/y)=w920:i32)  [unwired: 1 out]
                            n541 = Equal To 0?(x=w920) -> (x = 0?=w919:bool)
                            n542 = stacked-sequence {
                              seq-local: [_ w925 _ _] -> [_ _ w927 _]
                              tunnel: [_ w925 _ _] -> w923
                              tunnel: w919 -> [_ _ _ w929]
                              frame #0 {
                                "Pause message" <- "Measurement Program Paused!!!!" ("Pause message")
                              }
                              frame #1 {
                                n543 = global write "Trav_pos_global.vi" "Paused During Row?"(TRUE ("Paused During Row?")) -> ()
                                n544 = local read "Pause"() -> (w925:bool)
                              }
                              frame #2 {
                                n545 = property on="Pause message" class="Str"("Blinking"=w927, "Visible"=w927) -> ()  [unwired: 2 in, 2 out]
                                n546 = Wait Until Next ms Multiple(millisecond multiple=u32 1000) -> ()  [unwired: 1 out]
                              }
                              frame #3 {
                                n547 = case shown="True" w929 {
                                frame False {
                                }
                                frame True {
                                n548 = Current VI's Path() -> (path=w930:path)
                                n549 = call "Bring_to_front.vi"("path"=w930) -> ()
                                }
                                }
                              }
                            }
                          }
                        }
                        frame "Post Process Raw Data File" {
                          n550 = stacked-sequence {
                            seq-local: [_ w935 _] -> [_ _ w942]
                            tunnel: w932 -> [_ _ w943]
                            tunnel: [_ _ w941] -> w931
                            frame #0 {
                              n551 = local write "PP next block"(FALSE ("PP next block")) -> ()
                              n552 = property on="PP next block" class="Bool (strict)"("Visible"=TRUE) -> ()  [unwired: 2 in, 2 out]
                            }
                            frame #1 {
                              n553 = while {
                                tunnel: [w939] -> w935
                                stop <- w936 stop-if-true
                                n554 = local read "stop"() -> (w939:bool)
                                n555 = local read "Pause"() -> (w937:bool)
                                n556 = Compound Arithmetic op=OR(w939, "PP next block", invert w937) -> (w936:bool)
                                n557 = case shown="False" w936 {
                                frame False {
                                n558 = Wait (ms)(milliseconds to wait=u32 200) -> ()  [unwired: 1 out]
                                }
                                frame True {
                                }
                                }
                              }
                            }
                            frame #2 {
                              n559 = property on="PP next block" class="Bool (strict)"("Visible"=FALSE) -> ()  [unwired: 2 in, 2 out]
                              n560 = Or(x=w942, y=w943) -> (x .or. y?=w941:bool)
                            }
                          }
                        }
                      }
                    }
                  }
                }
              }
            }
          }
          frame Default {
            n561 = stacked-sequence {
              seq-local: [w953 _ _ _ _ _] -> [_ _ _ _ w1051 _]
              seq-local: [_ _ w963 _ _ _] -> [_ _ _ _ w1050 _]
              seq-local: [_ _ _ w1018 _ _] -> [_ _ _ _ w1049 _]
              seq-local: [_ w955 _ _ _ _] -> [_ _ _ _ w1048 _]
              seq-local: [_ _ w962 _ _ _] -> [_ _ _ w1017 _ _]
              frame #0 {
                n562 = Build Array("Name", "Index", "Channel", "Hz" ("element"), "Samples" ("element"), "Sync ms", "Max", "Min") -> (w953:string[])
              }
              frame #1 {
                n563 = global read "Meas_global.vi" "PWA Data"() -> (w956:T28)
                n564 = case shown="\"One Ch PWA\"" w956 {
                  tunnel: [string[][] [] w958] -> w955
                  frame "No PWA Data" {
                  }
                  frame "One Ch PWA" {
                    n565 = Build Array("PWA") -> (w959:string[])
                    n566 = Build Array(w959) -> (w958:string[][])
                  }
                }
              }
              frame #2 {
                n567 = global read "Meas_global.vi" "Analysis Info cluster"() -> (w964:T23[])
                n568 = global read "LDA_global.vi" "LDA Channels"() -> (w961:T29[])
                n569 = for {
                  tunnel: w964 -> [w966] mode=indexing
                  tunnel: [w972] -> w963 mode=indexing
                  tunnel: [w971] -> w962 mode=indexing
                  tunnel: w961 -> [w970]
                  i -> [w968]
                  n570 = Unbundle By Name(w966) -> ("chState"=w965:T24)
                  n571 = Index Array(array=w970, index=w968) -> (element=w969:T29)
                  n572 = Number To Decimal String(number=w968) -> (decimal integer string=w967:string)  [unwired: 1 in]
                  n573 = case shown="\"Mute\"" w965 {
                    tunnel: w966 -> [w977 w982]
                    tunnel: [w973 w981] -> w972
                    tunnel: [w974 w980] -> w971
                    tunnel: w969 -> [_ w979]
                    tunnel: w967 -> [_ w978]
                    frame "Mute" {
                      w975 = ""
                      n574 = Unbundle By Name(w977) -> ("Inst name"=w974:string)
                      n575 = Build Array(w974, "Muted" ("element"), w975, w975, w975, w975, w975, w975) -> (w973:string[])
                    }
                    frame Default {
                      n576 = stacked-sequence {
                        seq-local: [w987 _] -> [_ w1006]
                        seq-local: [w986 _] -> [_ w1005]
                        tunnel: w982 -> [w985 _]
                        tunnel: [_ w1004] -> w981
                        tunnel: [w983 _] -> w980
                        tunnel: w979 -> [_ w1003]
                        tunnel: w978 -> [w984 _]
                        frame #0 {
                          n577 = Unbundle By Name(w985) -> ("Inst name"=w983:string, "Ch No"=w1002:i16, "Req Sample Rate Hz"=w997:dbl, "Sync Delay Time (s)"=w990:dbl, "Inst Array"=w992:T20)
                          n578 = local read "Time per Block (s)"() -> (w999:dbl)
                          n579 = Equal?(x=w992, y=Instrument_Array."LDA" ("Inst Array")) -> (x = y?=w987:bool)
                          n580 = Multiply(x=w997, y=w999) -> (x*y=w998:dbl)
                          n581 = Multiply(x=w990, y=1000.0) -> (x*y=w989:dbl)
                          n582 = Number To Decimal String(number=w1002) -> (decimal integer string=w1001:string)  [unwired: 1 out]
                          n583 = Number To Decimal String(number=w998) -> (decimal integer string=w994:string)  [unwired: 1 out]
                          n584 = Number To Fractional String(number=w997, precision (6)=i16 1) -> (F-format string=w995:string)  [unwired: 2 in]
                          n585 = Format Into String(format string="%.1f" ("Format String"), w989) -> (resulting string=w993:string)  [unwired: 2 in, 1 out]
                          n586 = Build Array(w983, w984, w1001, w995, w994, w993) -> (w986:string[])
                        }
                        frame #1 {
                          n587 = case shown="True" w1006 {
                            tunnel: w1005 -> [w1007 w1014]
                            tunnel: [w1007 w1011] -> w1004
                            tunnel: w1003 -> [_ w1010]
                            frame False {
                            }
                            frame True {
                              n588 = Unbundle By Name(w1010) -> ("Max Velocity"=w1008:dbl, "Min Velocity"=w1009:dbl)
                              n589 = Format Into String(format string="%.1f m/s" ("Format String"), w1009) -> (resulting string=w1012:string)  [unwired: 2 in, 1 out]
                              n590 = Format Into String(format string="%.1f m/s" ("Format String"), w1008) -> (resulting string=w1013:string)  [unwired: 2 in, 1 out]
                              n591 = Build Array (concatenate)(w1014, w1013, w1012) -> (w1011:string[])
                            }
                          }
                        }
                      }
                    }
                  }
                }
              }
              frame #3 {
                n592 = global read "Meas_global.vi" "correlate"() -> (w1024:i32[][])
                n593 = for {
                  tunnel: w1024 -> [w1029] mode=indexing
                  tunnel: w1017 -> [w1028]
                  tunnel: "Correlating" -> [w1027]
                  tunnel: [w1025] -> w1019 mode=indexing
                  n594 = for {
                    tunnel: w1029 -> [w1032] mode=indexing
                    tunnel: w1028 -> [w1031]
                    tunnel: [w1030] -> w1026 mode=indexing
                    n595 = Index Array(array=w1031, index=w1032) -> (element=w1030:string)
                  }
                  n596 = Build Array (concatenate)(w1027, w1026) -> (w1025:string[])
                }
                n597 = Initialize Array("", 5 ("Dimension Size")) -> (w1020:string[])
                n598 = Build Array (concatenate)(w1020, w1019) -> (w1018:string[][])
              }
              frame #4 {
                w1036 = 0 ("index (row)")
                w1035 = 1 ("length")
                n599 = Build Array (concatenate)(w1051, w1048, w1050, w1049) -> (w1034:string[][])
                n600 = Array Size(array=w1034) -> (size(s)=w1047:i32[])
                n601 = Index Array(array=w1047) -> (element=w1046:i32)  [unwired: 1 in]
                n602 = Delete From Array(array=w1034, length=w1035, index (row)=w1036) -> (deleted portion=w1043:string[][], array with subset deleted=w1042:string[][])  [unwired: 1 in]
                n603 = Less?(x=w1046, y=16) -> (x < y?=w1045:bool)
                n604 = Delete From Array(array=w1042, length=w1035, index (col)=w1036) -> (deleted portion=w1041:string[][], array with subset deleted=w1033:string[][])  [unwired: 1 in]
                n605 = Index Array(array=w1043) -> (element=w1039:string[])  [unwired: 2 in]
                n606 = Index Array(array=w1041, index (col)=w1036) -> (element=w1040:string[])  [unwired: 1 in]
                n607 = case shown="True" w1045 {
                  frame False {
                  }
                  frame True {
                    n608 = property on="Statistics" class="Tbl (strict)"("Index Values"=T19 {"Row"=0, "Column"=0} ("Selection Start")) -> ()  [unwired: 2 in, 2 out]
                  }
                }
                n609 = Split 1D Array(array=w1039, index=1) -> (second subarray=w1038:string[])  [unwired: 1 out]
                n610 = property on="Statistics" class="Tbl (strict)"("Column Headers[]"=w1038, "Row Headers[]"=w1040) -> ()  [unwired: 2 in, 2 out]
                n611 = local write "Statistics"(w1033) -> ()
              }
              frame #5 {
                n612 = global read "Meas_global.vi" "Time Continuous Across Blocks"() -> (w1053:bool)
                n613 = Select(t="Continuous Time Trace", s=w1053, f="") -> (s? t:f=w1057:string)
                n614 = Build Array(w1057) -> (w1056:string[])
                n615 = Build Array(w1056) -> (w1055:string[][])
                n616 = Transpose 2D Array(2D array=w1055) -> (transposed array=w1054:string[][])
                n617 = local write "Diagnostic info"(w1054) -> ()
              }
            }
            n618 = global write "Meas_global.vi" "Current Block No"(1 ("Current Block No")) -> ()
          }
        }
      }
      frame #19 {
        n619 = global read "Meas_global.vi" "Raw data option"() -> (w1063:enum16{"Save raw data", "Raw data not saved"})
        n620 = global read "Meas_global.vi" "Post Process"() -> (w1062:T2)
        n621 = case shown="\"Save Current Setup\"" w1064 {
          tunnel: w1063 -> [w1068 _ _ _]
          tunnel: w1062 -> [w1067 _ w1105 w1108]
          tunnel: [w1066 w1089 w1104 w1107] -> w1061
          tunnel: i32[] [] -> [w1065 w1089 w1104 w1107]
          frame "Run Program" {
            n622 = case shown="\"Take New Data\"" w1067 {
              tunnel: w1068 -> [w1070 _]
              tunnel: [w1069 w1080] -> w1066
              tunnel: w1065 -> [w1069 w1079]
              frame "Take New Data" {
                n623 = case shown="\"Raw data not saved\"" w1070 {
                  frame "Save raw data" {
                  }
                  frame "Raw data not saved" {
                    n624 = global read "Meas_global.vi" "Remote control"() -> (w1073:bool)
                    n625 = case shown="False" w1073 {
                      tunnel: ["Current_Setup.xls" ("Setup filename") w1078] -> w1072
                      tunnel: [w1075 TRUE ("Measurement.vi Top level?")] -> w1071
                      frame False {
                        n626 = global read "Meas_global.vi" "Measurement.vi Top level?"() -> (w1075:bool)
                      }
                      frame True {
                        n627 = local read "Setup filename"() -> (w1078:string)
                      }
                    }
                    n628 = case shown="False" w1071 {
                      tunnel: w1072 -> [_ w1074]
                      frame False {
                      }
                      frame True {
                        n629 = call "Save_Setup_File.vi"("Setup filename"=w1074) -> ()  [unwired: 1 out]
                      }
                    }
                  }
                }
              }
              frame "Post Process Raw Data File" {
                n630 = global read "Meas_global.vi" "Pre Setup String"() -> (w1084:string)
                n631 = call "Get_Characters_from_string.vi"("Input string"=w1084, "Variable name"="Output no Stats for the following indices_(eg 0;5;7)") -> ("Value"=w1081:string)  [unwired: 1 in, 1 out]
                n632 = Empty String/Path?(string/path=w1081) -> (empty?=w1082:bool)
                n633 = case shown="True" w1082 {
                  tunnel: w1081 -> [w1087 _]
                  tunnel: [w1085 w1088] -> w1080
                  tunnel: w1079 -> [_ w1088]
                  frame False {
                    n634 = call "Get_array_values_fr_String.vi"("String Value"=w1087) -> ("Numeric Array"=w1086:dbl[])  [unwired: 1 out]
                    n635 = To Long Integer(number=w1086) -> (32bit integer=w1085:i32[])
                  }
                  frame True {
                  }
                }
              }
            }
          }
          frame "Save Current Setup" {
            n636 = stacked-sequence {
              seq-local: [w1092 _] -> [_ w1095]
              seq-local: [w1091 _] -> [_ w1094]
              frame #0 {
                w1093 = FALSE  # Save New File?
                n637 = call "Save_current_setup.vi"("Save New File?"=w1093, "Setup File Type"=Setup_Filetype."Measurement Setups") -> ("Cancelled?"=w1091:bool, "Saved filepath"=w1092:path)  [unwired: 1 in, 1 out]
              }
              frame #1 {
                n638 = case shown="False" w1094 {
                  tunnel: w1095 -> [w1096 _]
                  frame False {
                    n639 = stacked-sequence {
                      tunnel: w1096 -> [w1097 w1099]
                      frame #0 {
                        n640 = call "Input_Instrument_Positions.vi"("Filepath to Save"=w1097) -> ()  [unwired: 2 out]
                      }
                      frame #1 {
                        n641 = Strip Path(path=w1099) -> (stripped path=w1102:path)  [unwired: 1 out]
                        n642 = call "Create_setup_string.vi"() -> ("Setup String"=w1103:string)  [unwired: 1 out]
                        n643 = call "Add_length_to_string.vi"("String in"=w1103) -> ("String out"=w1098:string)
                        n644 = Build Path(base path=w1102, name or relative path="Current_Setup.xls") -> (appended path=w1100:path)
                        n645 = call "Write Characters with check.vi"("String to Write"=w1098, "file (use dialog)"=w1099) -> ()  [unwired: 2 in, 1 out]
                        n646 = call "Write Characters with check.vi"("String to Write"=w1098, "file (use dialog)"=w1100) -> ()  [unwired: 2 in, 1 out]
                      }
                    }
                  }
                  frame True {
                  }
                }
              }
            }
          }
          frame "Show Setup" {
            n647 = case shown="\"Take New Data\"" w1105 {
              frame "Take New Data" {
                n648 = call "Save_Setup_File.vi"("Setup filename"="Current_Setup.xls") -> ()  [unwired: 1 out]
              }
              frame "Post Process Raw Data File" {
              }
            }
          }
          frame "Setup Front Panel" {
            n649 = case shown="\"Take New Data\"" w1108 {
              frame "Take New Data" {
                n650 = stacked-sequence {
                  frame #0 {
                    n651 = global read "Trav_pos_global.vi" "Measurement setup files"() -> (w1110:string[])
                    n652 = Empty Array?(array=w1110) -> (empty?=w1109:bool)
                    n653 = case shown="False" w1109 {
                      frame False {
                        n654 = stacked-sequence {
                          frame #0 {
                            n655 = global read "Meas_global.vi" "Analysis Info cluster"() -> (w1112:T23[])
                            n656 = call "FFID Setup.vi"("Analysis Info cluster In"=w1112) -> ("Analysis Info cluster Out"=w1111:T23[])  [unwired: 9 in, 1 out]
                            n657 = global write "Meas_global.vi" "Analysis Info cluster"(w1111) -> ()
                          }
                          frame #1 {
                            n658 = local read "Setup filename"() -> (w1113:string)
                            n659 = call "Save_Setup_File.vi"("Setup filename"=w1113) -> ()  [unwired: 1 out]
                          }
                        }
                      }
                      frame True {
                      }
                    }
                  }
                  frame #1 {
                    n660 = Current VI's Path() -> (path=w1120:path)
                    n661 = global read "Meas_global.vi" "Acquisition_Plug_Ins to Run"() -> (w1119:string[])
                    n662 = Strip Path(path=w1120) -> (stripped path=w1114:path)  [unwired: 1 out]
                    n663 = Build Path(base path=w1114, name or relative path="Anemometry Sub Vis") -> (appended path=w1115:path)
                    n664 = Build Path(base path=w1115, name or relative path="Acquisition") -> (appended path=w1116:path)
                    n665 = Build Path(base path=w1116, name or relative path="Acquisition_Plug_Ins") -> (appended path=w1122:path)
                    n666 = for {
                      tunnel: w1122 -> [w1132]
                      tunnel: w1119 -> [w1125] mode=indexing
                      n667 = Build Path(base path=w1132, name or relative path=w1125) -> (appended path=w1127:path)
                      n668 = Open VI Reference(type specifier VI Refnum (for type only)=refnum<vi> refnum, vi path=w1127) -> (vi reference=w1128:refnum<vi>, error out=w1129:errorcluster)  [unwired: 4 in]
                      n669 = Concatenate Strings(w1125, " Port Error" ("string")) -> (w1123:string)
                      n670 = call-by-ref "?"(reference=w1128, error in=w1129) -> (reference out=w1131:refnum<vi>, error out=w1130:errorcluster, "error out"=w1126:errorcluster)  [unwired: 1 in]
                      n671 = Close Reference(reference=w1131, error in (no error)=w1130) -> ()  [unwired: 1 out]
                      n672 = call "EnFlo_Error_Handler.vi"("error in (no error)"=w1126, "Error Type"=w1123) -> ()  [unwired: 2 in, 2 out]
                    }
                  }
                }
              }
              frame "Post Process Raw Data File" {
              }
            }
          }
        }
        n673 = global write "Meas_global.vi" "Blank Output Stats for Chs"(w1061) -> ()
      }
      frame #20 {
        n674 = global read "Meas_global.vi" "Duplicate_Channels_by_Arithmetic"() -> (w1136:i32[][])
        n675 = Array Size(array=w1136) -> (size(s)=w1137:i32[])
        n676 = Index Array(array=w1137) -> (element=w1135:i32)  [unwired: 1 in]
        n677 = Greater Than 0?(x=w1135) -> (x > 0?=w1134:bool)
        n678 = case shown="True" w1134 {
          tunnel: w1136 -> [_ w1138]
          frame False {
          }
          frame True {
            n679 = global read "Meas_global.vi" "Analysis Info cluster"() -> (w1140:T23[])
            n680 = for {
              tunnel: w1140 -> [w1158]
              tunnel: w1138 -> [w1157] mode=indexing
              shift-right: [w1152] -> w1139
              shift-left: w1140 -> [w1153]
              n681 = Index Array(array=w1157) -> (element #1=w1156:i32, element #2=w1154:i32)  [unwired: 2 in]
              n682 = Index Array(array=w1158, index=w1156) -> (element=w1155:T23)
              n683 = Unbundle By Name(w1155) -> ("Inst name"=w1150:string, "U"=w1145:dbl, "u^2"=w1144:dbl)
              n684 = Concatenate Strings(w1150, ":Mean:" ("string")) -> (w1147:string)
              n685 = Concatenate Strings(w1150, ":Variance:" ("string")) -> (w1148:string)
              n686 = call "Number_2_string.vi"("number"=w1145) -> ("String"=w1143:string)  [unwired: 1 in]
              n687 = call "Number_2_string.vi"("number"=w1144) -> ("String"=w1142:string)  [unwired: 1 in]
              n688 = Build Array(w1147, w1148) -> (w1146:string[])
              n689 = Build Array(w1143, w1142) -> (w1141:string[])
              n690 = in-place {
                in-place-border: w1146 -> [w1160]
                in-place-border: w1141 -> [w1159]
                n691 = in-place-array #2(w1153, w1154) -> (w1162:T23)
                n692 = call "Update Metadata channels.vi"("Metadata Values"=w1159, "Metadata Names"=w1160, "Analysis info Cluster in"=w1162) -> ("Analysis info Cluster out"=w1161:T23)
                n693 = in-place-array #2(w1161) -> (w1152:T23[])  [unwired: 1 out]
              }
            }
            n694 = global write "Meas_global.vi" "Analysis Info cluster"(w1139) -> ()
          }
        }
      }
      frame #21 {
        n695 = global read "Meas_global.vi" "Duplicate Chs to correlate"() -> (w1165:i32[][])
        n696 = Array Size(array=w1165) -> (size(s)=w1166:i32[])
        n697 = Index Array(array=w1166) -> (element=w1163:i32)  [unwired: 1 in]
        n698 = Greater Than 0?(x=w1163) -> (x > 0?=w1164:bool)
        n699 = case shown="True" w1164 {
          tunnel: w1165 -> [_ w1167]
          frame False {
          }
          frame True {
            n700 = global read "Meas_global.vi" "correlate"() -> (w1171:i32[][])
            n701 = global read "Meas_global.vi" "Correlation Results"() -> (w1169:T30[])
            n702 = Array Size(array=w1171) -> (size(s)=w1172:i32[])
            n703 = global read "Meas_global.vi" "Analysis Info cluster"() -> (w1174:T23[])
            n704 = Index Array(array=w1172) -> (element=w1170:i32)  [unwired: 1 in]
            n705 = Array Subset(array=w1169, index=w1170) -> (w1168:T30[])  [unwired: 1 in]
            n706 = for {
              shift-right: [w1194] -> w1173
              shift-left: w1174 -> [w1179]
              tunnel: w1168 -> [w1183] mode=indexing
              tunnel: w1167 -> [w1182] mode=indexing
              n707 = Unbundle By Name(w1183) -> ("U inst"=w1176:string, "W inst"=w1175:string, "uw"=w1188:dbl, "uw/u'w'"=w1187:dbl)
              n708 = Index Array(array=w1182, index=2) -> (element=w1181:i32)
              n709 = call "Number_2_string.vi"("number"=w1188) -> ("String"=w1186:string)  [unwired: 1 in]
              n710 = call "Number_2_string.vi"("number"=w1187) -> ("String"=w1185:string)  [unwired: 1 in]
              n711 = Format Into String(format string="%s:%s:", w1176, w1175) -> (resulting string=w1177:string)  [unwired: 2 in, 1 out]
              n712 = Concatenate Strings(w1177, "Correlation" ("string")) -> (w1190:string)
              n713 = Concatenate Strings(w1177, "Corr_Coeff" ("string")) -> (w1191:string)
              n714 = Build Array(w1190, w1191) -> (w1189:string[])
              n715 = Build Array(w1186, w1185) -> (w1184:string[])
              n716 = in-place {
                in-place-border: w1189 -> [w1196]
                in-place-border: w1184 -> [w1195]
                n717 = in-place-array #3(w1179, w1181) -> (w1198:T23)
                n718 = call "Update Metadata channels.vi"("Metadata Values"=w1195, "Metadata Names"=w1196, "Analysis info Cluster in"=w1198) -> ("Analysis info Cluster out"=w1197:T23)
                n719 = in-place-array #3(w1197) -> (w1194:T23[])  [unwired: 1 out]
              }
            }
            n720 = global write "Meas_global.vi" "Analysis Info cluster"(w1173) -> ()
          }
        }
      }
      frame #22 {
        n721 = case shown="\"Run Program\"" w1200 {
          tunnel: w1200 -> [w1204 _ _ _]
          tunnel: [w1204 w1217 w1218 w1219] -> w1199
          frame "Run Program" {
            n722 = global read "Meas_global.vi" "Analysis Info cluster"() -> (w1203:T23[])
            n723 = for {
              tunnel: w1203 -> [w1215] mode=indexing
              stop <- w1205 stop-if-true
              w1212 = "Pitot ("
              n724 = Unbundle By Name(w1215) -> ("U"=w1206:dbl, "Inst name"=w1211:string)
              n725 = String Length(string=w1212) -> (length=w1214:i32)
              n726 = String Subset(string=w1211, length (rest)=w1214) -> (substring=w1213:string)  [unwired: 1 out]
              n727 = Equal?(x=w1213, y=w1212) -> (x = y?=w1208:bool)
              n728 = call "Match_Pat_Case_In.vi"("String to match"="ref", "String"=w1211) -> ("offset past match"=w1209:i32)  [unwired: 1 in, 3 out]
              n729 = Greater Or Equal To 0?(x=w1209) -> (x >= 0?=w1207:bool)
              n730 = And(x=w1207, y=w1208) -> (x .and. y?=w1205:bool)
              n731 = case shown="True" w1205 {
                tunnel: w1206 -> [_ w1216]
                frame False {
                }
                frame True {
                  n732 = call "Log_Reference_Velocity.vi"("Measured Velocity"=w1216) -> ()  [unwired: 1 out]
                }
              }
            }
          }
          frame "Show Setup" {
            w1217 = Setup."Run Program"  # setup
          }
          frame "Save Current Setup" {
            w1218 = Setup."Run Program"  # setup
          }
          frame "Setup Front Panel" {
            w1219 = Setup."Run Program"  # setup
          }
        }
        n733 = local read "Correlate?"() -> (w1202:T8)
        n734 = case shown="\"Cross correlation off\"" w1202 {
          tunnel: [T8."Cross correlation off" T8."Correlate without activating panel" T8."Correlate without activating panel"] -> w1201
          frame "Cross correlation off" {
          }
          frame "Show correlation panel" {
          }
          frame "Correlate without activating panel" {
          }
        }
        n735 = local write "Correlate?"(w1201) -> ()
        n736 = local write "setup"(w1199) -> ()
      }
      frame #23 {
        n737 = global read "Dynamic_call_global.ph.vi" "Initial Plug Ins"() -> (w1227:string[])
        n738 = case shown="\"Run Program\"" w1229 {
          frame "Run Program" {
            n739 = global read "Dynamic_call_global.ph.vi" "Final Plug Ins"() -> (w1258:string[])
            n740 = call "Plug_in_Directories.vi"() -> ("Final"=w1257:path)  [unwired: 2 in, 4 out]
            n741 = for {
              tunnel: w1258 -> [w1263] mode=indexing
              tunnel: w1257 -> [w1262]
              tunnel: [w1260] -> w1252 mode=concatenating
              tunnel: [w1259] -> w1251 mode=concatenating
              w1266 = FALSE  # Dialog Box (T)
              n742 = Build Path(base path=w1262, name or relative path=w1263) -> (appended path=w1261:path)
              n743 = global read "Dynamic_call_global.ph.vi" "Plug in"() -> (w1271:refnum<vi>)
              n744 = Open VI Reference(type specifier VI Refnum (for type only)=w1271, vi path=w1261) -> (vi reference=w1270:refnum<vi>, error out=w1269:errorcluster)  [unwired: 2 in, 2 out]
              n745 = call-by-ref "?"(reference=w1270, error in=w1269) -> (reference out=w1267:refnum<vi>, error out=w1268:errorcluster, "Plug in titles"=w1260:string[], "Plug in values"=w1259:string[])  [unwired: 6 in]
              n746 = Close Reference(reference=w1267, error in (no error)=w1268) -> (error out=w1264:errorcluster)
              n747 = call "EnFlo_Error_Handler.vi"("error in (no error)"=w1264, "Error Type"="Running Final Plug In", "Dialog Box (F)"=w1266) -> ()  [unwired: 3 out]
            }
            n748 = global read "Dynamic_call_global.ph.vi" "Plug in values"() -> (w1253:string[])
            n749 = global read "Dynamic_call_global.ph.vi" "Plug in titles"() -> (w1254:string[])
            n750 = Build Array (concatenate)(w1254, w1252) -> (w1256:string[])
            n751 = Build Array (concatenate)(w1253, w1251) -> (w1255:string[])
            n752 = global write "Dynamic_call_global.ph.vi" "Plug in titles"(w1256) -> ()
            n753 = global write "Dynamic_call_global.ph.vi" "Plug in values"(w1255) -> ()
          }
          frame "Show Setup", Default {
          }
        }
        n754 = Search 1D Array(1D array=w1227, element="Puff_using_Arduino.vi") -> (index of element=w1226:i32)  [unwired: 1 in]
        n755 = Less Than 0?(x=w1226) -> (x < 0?=w1224:bool)
        n756 = And(x=w1224, y=w1225) -> (x .and. y?=w1223:bool)
        n757 = case shown="True" w1223 {
          frame False {
          }
          frame True {
            n758 = global read "Meas_global.vi" "Analysis Info cluster"() -> (w1232:T23[])
            n759 = for {
              tunnel: w1232 -> [w1250] mode=indexing
              tunnel: [w1244] -> w1230 mode=concatenating if=w1247
              n760 = Unbundle By Name(w1250) -> ("Inst name"=w1246:string, "Point Drift"=w1243:dbl)
              n761 = Multiply(x=100.0, y=w1243) -> (x*y=w1241:dbl)
              n762 = Absolute Value(x=w1243) -> (abs(x)=w1249:dbl)
              n763 = Format Into String(format string="%s = %.1f%%\\n", w1246, w1241) -> (resulting string=w1244:string)  [unwired: 2 in, 1 out]
              n764 = Greater?(x=w1249, y=1.0) -> (0:w1247:bool)
            }
            n765 = Empty String/Path?(string/path=w1230) -> (empty?=w1231:bool)
            n766 = case shown="False" w1231 {
              tunnel: w1230 -> [w1237 _]
              frame False {
                w1240 = FALSE  # Dialog Box (T)
                n767 = Concatenate Strings("List of Instrument whose standard deviation is changed by more 100% by removing the drift in the time trace:\n", w1237) -> (w1234:string)
                n768 = Bundle By Name(cluster=errorcluster {"status"=FALSE, "code"=0, "source"=""} ("error out"), "status"=TRUE, "source"=w1234) -> (w1233:errorcluster)
                n769 = call "EnFlo_Error_Handler.vi"("error in (no error)"=w1233, "Error Type"="Unsteady Point", "Dialog Box (F)"=w1240) -> ()  [unwired: 3 out]
              }
              frame True {
              }
            }
          }
        }
      }
      frame #24 {
        n770 = global read "Meas_global.vi" "Post Process"() -> (w1277:T2)
        n771 = global read "Meas_global.vi" "Repeat Measurement?"() -> (w1272:bool)
        n772 = Equal?(x=w1277, y=Post_Process."Take New Data" ("Post Process")) -> (x = y?=w1275:bool)
        n773 = Equal?(x=w1278, y=Setup."Run Program" ("setup")) -> (x = y?=w1274:bool)
        n774 = Compound Arithmetic op=AND(invert w1272, w1274, w1275) -> (w1273:bool)
        n775 = local read "stop"() -> (w1282:bool)
        n776 = case shown="False" w1282 {
          tunnel: [w1294 Multi_Run_Status."Terminate Run" ("Status Out")] -> w1281
          frame False {
            n777 = global read "Meas_global.vi" "Status"() -> (w1294:T1)
          }
          frame True {
          }
        }
        n778 = case shown="True" w1273 {
          tunnel: w1281 -> [w1283 w1287]
          tunnel: [w1283 w1288] -> w1280
          frame False {
          }
          frame True {
            n779 = local read "Raw data file"() -> (w1284:path)
            n780 = Path to Array of Strings(0:w1284) -> (2:w1289:string[])  [unwired: 1 out]
            n781 = Index Array(array=w1289, index=0 ("Index")) -> (element=w1286:string)
            n782 = Build Array(w1286) -> (w1285:string[])
            n783 = for {
              tunnel: w1285 -> [w1293] mode=indexing
              shift-right: [w1291] -> w1288
              shift-left: w1287 -> [w1292]
              n784 = call "Warn_on_low_HD_space.vi"("Status In"=w1292, "HD name"=w1293) -> ("Status Out"=w1291:T1)  [unwired: 6 out]
            }
          }
        }
        "Status Out" <- w1280
      }
      frame #25 {
        # "Results are written here"
        n785 = global read "Meas_global.vi" "Repeat Measurement?"() -> (w1300:bool)
        n786 = global read "Meas_global.vi" "MeasurementStartTime"() -> (w1296:dbl)
        n787 = global read "Meas_global.vi" "File"() -> (w1302:T15)
        n788 = Equal?(x=Setup."Run Program" ("setup"), y=w1307) -> (x = y?=w1305:bool)
        n789 = Not Equal?(x=w1302, y=T15."Save no data" ("File")) -> (x != y?=w1306:bool)
        n790 = Compound Arithmetic op=AND(w1305, w1306) -> (w1304:bool)
        n791 = local read "Setup filename"() -> (w1299:string)
        n792 = Get Date/Time In Seconds() -> (seconds since 1Jan1904=w1298:timestamp)
        n793 = To Double Precision Float(number=w1298) -> (double precision float=w1297:dbl)
        n794 = case shown="False" w1300 {
          tunnel: w1304 -> [w1311 _]
          tunnel: w1296 -> [w1310 _]
          tunnel: w1299 -> [w1309 _]
          tunnel: w1297 -> [w1308 _]
          frame False {
            n795 = case shown="False" w1311 {
              tunnel: w1308 -> [w1314 w1350]
              tunnel: w1309 -> [w1313 w1349]
              tunnel: w1310 -> [w1312 w1348]
              frame True {
                n796 = stacked-sequence {
                  seq-local: [_ w1322 _] -> [_ _ w1341]
                  tunnel: w1314 -> [w1315 _ _]
                  tunnel: w1313 -> [w1317 _ _]
                  tunnel: w1312 -> [w1316 _ _]
                  frame #0 {
                    n797 = global write "Meas_global.vi" "MeasurementEndTime"(w1315) -> ()
                    n798 = call "Write_Results_file.vi"("Experiment start time"=w1316, "Experiment End time"=w1315, "Setup filename"=w1317) -> ()  [unwired: 4 out]
                  }
                  frame #1 {
                    n799 = global read "Meas_global.vi" "Raw data file"() -> (w1328:path)
                    n800 = global read "Trav_pos_global.vi" "Top level setup filename"() -> (w1326:path)
                    n801 = global read "Meas_global.vi" "Start Time of experiment"() -> (w1325:dbl)
                    n802 = Strip Path(path=w1328) -> (stripped path=w1318:path)  [unwired: 1 out]
                    n803 = Strip Path(path=w1318) -> (stripped path=w1323:path)  [unwired: 1 out]
                    n804 = Empty String/Path?(string/path=w1326) -> (empty?=w1327:bool)
                    n805 = Build Path(base path=w1323, name or relative path="Extra Info") -> (appended path=w1322:path)
                    n806 = case shown="False" w1327 {
                      tunnel: w1326 -> [w1340 _]
                      tunnel: w1325 -> [w1337 _]
                      tunnel: w1322 -> [w1333 _]
                      frame False {
                        n807 = call "Sec_to_date_filename.vi"("ss1904"=w1337) -> ("YYYY-mm-DD HH:MM"=w1332:string)  [unwired: 5 in, 9 out]
                        n808 = Format Into String(format string="Cmd_%s.xls", w1332) -> (resulting string=w1335:string)  [unwired: 2 in, 1 out]
                        n809 = call "Fast_string_Replace.vi"("Replace match with:"="-", "Input String"=w1335, "matchThis"=":" ("regular expression")) -> ("Output String"=w1331:string)  [unwired: 1 in, 1 out]
                        n810 = Build Path(base path=w1333, name or relative path=w1331) -> (appended path=w1338:path)
                        n811 = Copy(10:w1338, 11:w1340) -> ()  [unwired: 1 in, 5 out]
                      }
                      frame True {
                      }
                    }
                    n812 = global read "Meas_global.vi" "Post Process"() -> (w1321:T2)
                    n813 = Equal?(x=w1321, y=Post_Process."Take New Data" ("Post Process")) -> (x = y?=w1319:bool)
                    n814 = case shown="True" w1319 {
                      tunnel: w1318 -> [_ w1329]
                      frame False {
                      }
                      frame True {
                        w1330 = FALSE  # Empty list
                        n815 = call "Remember_RD_Folders.vi"("Empty list"=w1330, "Folders to Remember"=w1329) -> ()  [unwired: 1 out]
                      }
                    }
                  }
                  frame #2 {
                    n816 = global read "Meas_global.vi" "LDA data"() -> (w1342:enum16{"No LDA data", "Take LDA data"})
                    n817 = case shown="\"Take LDA data\"" w1342 {
                      tunnel: w1341 -> [_ w1346]
                      frame "No LDA data" {
                      }
                      frame "Take LDA data" {
                        w1344 = "LDA_Probe_Orientation.txt" ("name or relative path")
                        n818 = call "Setup_Filepath.vi"("Setup File Type"=Setup_Filetype."General", "Filename in"=w1344) -> ("Filename Out"=w1343:path)  [unwired: 1 out]
                        n819 = Build Path(base path=w1346, name or relative path=w1344) -> (appended path=w1347:path)
                        n820 = Copy(10:w1347, 11:w1343) -> ()  [unwired: 1 in, 5 out]
                      }
                    }
                  }
                }
              }
              frame False {
                n821 = global read "Meas_global.vi" "Raw data option"() -> (w1351:enum16{"Save raw data", "Raw data not saved"})
                n822 = case shown="\"Save raw data\"" w1351 {
                  tunnel: w1348 -> [w1354 _]
                  tunnel: w1350 -> [w1353 _]
                  tunnel: w1349 -> [w1352 _]
                  frame "Save raw data" {
                    n823 = stacked-sequence {
                      tunnel: w1354 -> [_ w1364]
                      tunnel: w1353 -> [_ w1363]
                      tunnel: w1352 -> [_ w1361]
                      frame #0 {
                        n824 = global read "Meas_global.vi" "Current Block No"() -> (w1355:i32)
                        n825 = global write "Meas_global.vi" "Requested No of blocks"(w1355) -> ()
                      }
                      frame #1 {
                        n826 = call "Create_Raw_data_file.vi"("Setup filename"=w1361, "Start time"=w1364, "End time"=w1363, "No of averages"=1) -> ("Column headers"=w1357:string[], "Values"=w1360:string[][])  [unwired: 2 in, 1 out]
                        n827 = for {
                          tunnel: w1357 -> [w1367] mode=indexing
                          tunnel: [w1365] -> w1356 mode=indexing
                          n828 = Match Pattern(string=w1367, regular expression=":") -> (after substring=w1365:string)  [unwired: 1 in, 3 out]
                        }
                        n829 = Index Array(array=w1360, index (row)=0) -> (element=w1358:string[])  [unwired: 1 in]
                        n830 = global write "Dynamic_call_global.ph.vi" "Plug in values"(w1358) -> ()
                        n831 = global write "Dynamic_call_global.ph.vi" "Plug in titles"(w1356) -> ()
                      }
                    }
                  }
                  frame "Raw data not saved" {
                  }
                }
              }
            }
          }
          frame True {
          }
        }
      }
      frame #26 {
        n832 = stacked-sequence {
          seq-local: [w1376 _] -> [_ w1381]
          seq-local: [w1370 _] -> [_ w1380]
          tunnel: w1368 -> [w1379 _]
          frame #0 {
            n833 = global read "Meas_global.vi" "Raw data file"() -> (w1374:path)
            n834 = global read "Meas_global.vi" "Raw data option"() -> (w1378:enum16{"Save raw data", "Raw data not saved"})
            n835 = Equal?(x=Setup."Run Program" ("setup"), y=w1379) -> (x = y?=w1373:bool)
            n836 = Strip Path(path=w1374) -> (stripped path=w1371:path)  [unwired: 1 out]
            n837 = Equal?(x=w1378, y=enum16{"Save raw data", "Raw data not saved"}."Save raw data" ("Raw data option")) -> (x = y?=w1372:bool)
            n838 = Strip Path(path=w1371) -> (stripped path=w1370:path)  [unwired: 1 out]
            n839 = global read "Meas_global.vi" "Repeat Measurement?"() -> (w1369:bool)
            n840 = Compound Arithmetic op=AND(invert w1369, w1373, w1372) -> (w1376:bool)
          }
          frame #1 {
            n841 = case shown="True" w1381 {
              tunnel: w1380 -> [_ w1382]
              frame False {
              }
              frame True {
                n842 = stacked-sequence {
                  seq-local: [_ _ w1422 _] -> [_ _ _ w1436]
                  tunnel: w1382 -> [w1383 w1411 w1423 _]
                  frame #0 {
                    n843 = global read "Trav_pos_global.vi" "Traverses to Move"() -> (w1385:string[])
                    n844 = global read "Constants_global.vi" "Traverse folder"() -> (w1386:path)
                    n845 = for {
                      tunnel: w1386 -> [w1399]
                      tunnel: w1385 -> [w1395] mode=indexing
                      tunnel: w1383 -> [w1396]
                      tunnel: string[] ["Traverse_Preferences.txt", "Traverse_Setup.xls"] ("Traverses to Move") -> [w1389]
                      n846 = Build Path(base path=w1399, name or relative path=w1395) -> (appended path=w1392:path)
                      n847 = Build Path(base path=w1392, name or relative path="Trav_Space_Files" ("Substring")) -> (appended path=w1398:path)
                      n848 = Build Path(base path=w1398, name or relative path="Selected_Filename.txt" ("Substring")) -> (appended path=w1402:path)
                      n849 = call "Create_directory_path.vi"("Path name"=w1402) -> ("Path name Out"=w1388:path)  [unwired: 2 in, 1 out]
                      n850 = Build Path(base path=w1396, name or relative path=w1395) -> (appended path=w1391:path)
                      n851 = for {
                        tunnel: w1392 -> [w1409]
                        tunnel: w1391 -> [w1407]
                        tunnel: w1389 -> [w1405] mode=indexing
                        n852 = Build Path(base path=w1409, name or relative path=w1405) -> (appended path=w1408:path)
                        n853 = Build Path(base path=w1407, name or relative path=w1405) -> (appended path=w1404:path)
                        n854 = call "Create_directory_path.vi"("Path name"=w1404) -> ("Path name Out"=w1403:path)  [unwired: 2 in, 1 out]
                        n855 = Copy(9:TRUE ("overwrite (F)"), 10:w1403, 11:w1408) -> ()  [unwired: 2 in, 3 out]
                      }
                      n856 = call "Read Characters with check.vi"("file (use dialog)"=w1388) -> ("Read String"=w1387:string)  [unwired: 1 in, 1 out]
                      n857 = Build Path(base path=w1391, name or relative path=w1387) -> (appended path=w1394:path)
                      n858 = Build Path(base path=w1398, name or relative path=w1387) -> (appended path=w1397:path)
                      n859 = call "Create_directory_path.vi"("Path name"=w1394) -> ("Path name Out"=w1393:path)  [unwired: 2 in, 1 out]
                      n860 = Copy(9:TRUE ("overwrite (F)"), 10:w1393, 11:w1397) -> ()  [unwired: 2 in, 3 out]
                    }
                  }
                  frame #1 {
                    n861 = local read "Setup filename"() -> (w1410:string)
                    n862 = Build Path(base path=w1411, name or relative path="Measurement_Setups") -> (appended path=w1413:path)
                    n863 = Build Path(base path=w1413, name or relative path=w1410) -> (appended path=w1412:path)
                    n864 = call "Does_file_exist_(simple).vi"("Pathname"=w1412) -> ("exists?"=w1415:bool)
                    n865 = case shown="False" w1415 {
                      tunnel: w1412 -> [w1417 _]
                      tunnel: w1410 -> [w1418 _]
                      frame False {
                        n866 = call "Create_directory_path.vi"("Path name"=w1417) -> ("Path name Out"=w1416:path)  [unwired: 2 in, 1 out]
                        n867 = call "Setup_Filepath.vi"("Setup File Type"=Setup_Filetype."Measurement Setups", "Filename in"=w1418) -> ("Filename Out"=w1419:path)  [unwired: 1 out]
                        n868 = Copy(9:TRUE ("overwrite (F)"), 10:w1416, 11:w1419) -> ()  [unwired: 2 in, 3 out]
                      }
                      frame True {
                      }
                    }
                  }
                  frame #2 {
                    n869 = global read "Meas_global.vi" "LDA data"() -> (w1425:enum16{"No LDA data", "Take LDA data"})
                    n870 = Build Path(base path=w1423, name or relative path="Extra Info") -> (appended path=w1422:path)
                    n871 = case shown="\"Take LDA data\"" w1425 {
                      tunnel: w1422 -> [_ w1426]
                      frame "No LDA data", Default {
                      }
                      frame "Take LDA data" {
                        w1427 = "Beam_Check_Positions.xls" ("Substring")
                        n872 = Build Path(base path=w1426, name or relative path=w1427) -> (appended path=w1428:path)
                        n873 = call "Does_file_exist_(simple).vi"("Pathname"=w1428) -> ("exists?"=w1429:bool)
                        n874 = case shown="False" w1429 {
                          tunnel: w1428 -> [w1434 _]
                          tunnel: w1427 -> [w1431 _]
                          frame False {
                            n875 = global read "Constants_global.vi" "All_Users"() -> (w1432:path)
                            n876 = call "Create_directory_path.vi"("Path name"=w1434) -> ("Path name Out"=w1433:path)  [unwired: 2 in, 1 out]
                            n877 = Build Path(base path=w1432, name or relative path=w1431) -> (appended path=w1430:path)
                            n878 = Copy(9:TRUE ("overwrite (F)"), 10:w1433, 11:w1430) -> ()  [unwired: 2 in, 3 out]
                          }
                          frame True {
                          }
                        }
                      }
                    }
                  }
                  frame #3 {
                    n879 = global read "Meas_global.vi" "Zero Offsetting filename"() -> (w1437:string)
                    n880 = Empty String/Path?(string/path=w1437) -> (empty?=w1438:bool)
                    n881 = case shown="False" w1438 {
                      tunnel: w1437 -> [w1440 _]
                      tunnel: w1436 -> [w1439 _]
                      frame False {
                        n882 = Build Path(base path=w1439, name or relative path=w1440) -> (appended path=w1441:path)
                        n883 = call "Does_file_exist_(simple).vi"("Pathname"=w1441) -> ("exists?"=w1442:bool)
                        n884 = case shown="False" w1442 {
                          tunnel: w1441 -> [w1446 _]
                          tunnel: w1440 -> [w1444 _]
                          frame False {
                            n885 = call "Get Calib Filepath.vi"("Filename String"=w1444) -> ("Filename Out"=w1443:path)  [unwired: 2 in]
                            n886 = call "Create_directory_path.vi"("Path name"=w1446) -> ("Path name Out"=w1445:path)  [unwired: 2 in, 1 out]
                            n887 = Copy(9:TRUE ("overwrite (F)"), 10:w1445, 11:w1443) -> ()  [unwired: 2 in, 3 out]
                          }
                          frame True {
                          }
                        }
                      }
                      frame True {
                      }
                    }
                  }
                }
              }
            }
          }
        }
      }
      frame #27 {
        n888 = global read "Meas_global.vi" "Repeat Measurement?"() -> (w1448:bool)
        n889 = global read "Meas_global.vi" "Post Process"() -> (w1457:T2)
        n890 = global read "Meas_global.vi" "LDA data"() -> (w1456:enum16{"No LDA data", "Take LDA data"})
        n891 = Equal?(x=Setup."Run Program" ("setup"), y=w1451) -> (x = y?=w1450:bool)
        n892 = Equal?(x=w1456, y=enum16{"No LDA data", "Take LDA data"}."Take LDA data" ("LDA data")) -> (x = y?=w1454:bool)
        n893 = Equal?(x=w1457, y=Post_Process."Take New Data" ("Post Process")) -> (x = y?=w1449:bool)
        n894 = case shown="False" w1448 {
          tunnel: w1449 -> [_ w1466]
          frame False {
            w1463 = FALSE  # Dialog Box (T)
            n895 = global read "Meas_global.vi" "Over/Under string"() -> (w1461:string)
            n896 = Empty String/Path?(string/path=w1461) -> (empty?=w1460:bool)
            n897 = Not(x=w1460) -> (.not. x?=w1459:bool)
            n898 = Bundle By Name(cluster=errorcluster {"status"=FALSE, "code"=0, "source"=""} ("error in (no error)"), "source"=w1461, "status"=w1459) -> (w1464:errorcluster)
            n899 = call "EnFlo_Error_Handler.vi"("error in (no error)"=w1464, "Error Type"="Signal Clipping", "Dialog Box (F)"=w1463) -> ()  [unwired: 3 out]
          }
          frame True {
            n900 = case shown="True" w1466 {
              frame False {
              }
              frame True {
                n901 = global read "Meas_global.vi" "Raw data file"() -> (w1467:path)
                n902 = Delete(path (use dialog)=w1467) -> ()  [unwired: 4 in, 3 out]
              }
            }
          }
        }
        n903 = Compound Arithmetic op=AND(invert w1448, w1450, w1449, w1454) -> (w1453:bool)
        n904 = case shown="False" w1453 {
          frame False {
          }
          frame True {
            n905 = call "Check LDA Data Rate.vi"() -> ()  [unwired: 12 in]
          }
        }
      }
      frame #28 {
        n906 = global read "Meas_global.vi" "Repeat Measurement?"() -> (w1475:bool)
        n907 = Empty String/Path?(string/path=w1468) -> (empty?=w1469:bool)
        n908 = case shown="False" w1469 {
          tunnel: w1468 -> [w1481 _]
          frame False {
            # "Scrub comments from MR"
            n909 = local read "Comments"() -> (w1480:string)
            n910 = call "Fast_string_Replace.vi"("Replace match with:"="", "Input String"=w1480, "matchThis"=w1481) -> ("Output String"=w1478:string)  [unwired: 1 in, 1 out]
            n911 = global write "Meas_global.vi" "Comments"(w1478) -> ()
            n912 = local write "Comments"(w1478) -> ()
          }
          frame True {
          }
        }
        n913 = case shown="True" w1475 {
          tunnel: w1477 -> [_ w1498]
          tunnel: [FALSE w1496] -> w1476
          frame False {
            n914 = global read "Meas_global.vi" "Error Messages"() -> (w1486:string)
            n915 = Empty String/Path?(string/path=w1486) -> (empty?=w1487:bool)
            n916 = case shown="False" w1487 {
              tunnel: w1486 -> [w1490 _]
              frame False {
                n917 = Bundle By Name(cluster=errorcluster {"status"=FALSE, "code"=0, "source"=""} ("error in (no error)"), "status"=TRUE, "source"=w1490) -> (w1492:errorcluster)
                n918 = global write "Meas_global.vi" "Error Messages"("") -> ()
                n919 = call "EnFlo_Error_Handler.vi"("error in (no error)"=w1492, "Dialog Box (F)"=FALSE ("Dialog Box (T)")) -> ()  [unwired: 1 in, 3 out]
              }
              frame True {
              }
            }
          }
          frame True {
            n920 = local read "stop"() -> (w1495:bool)
            n921 = Equal To 0?(x=w1498) -> (x = 0?=w1497:bool)
            n922 = Compound Arithmetic op=AND(invert w1495, w1497) -> (w1496:bool)
          }
        }
        n923 = global write "Meas_global.vi" "Files to Update"(T22[] [] ("Files to Update")) -> ()
        n924 = global write "Trav_pos_global.vi" "Dummy Measurement?"(FALSE ("Dummy Measurement?")) -> ()
        n925 = global write "Meas_global.vi" "Extra Comments"("") -> ()
        n926 = global write "Meas_global.vi" "Actual Measurement time (min)"(0.0 ("Max Measurement time (min)")) -> ()
        n927 = case shown="False" w1476 {
          frame False {
            w1485 = string[] [] ("Per Block Plug Ins Extra")
            n928 = global write "Meas_global.vi" "Delay before taking data (ms)"(u32 0 ("Delay before taking data (ms)")) -> ()
            n929 = global write "Plug_in_data_global.vi" "Server Channels to log"(string[] [] ("Server Channels to log")) -> ()
            n930 = global write "Dynamic_call_global.ph.vi" "Per Block Plug Ins Extra"(w1485) -> ()
            n931 = global write "Meas_global.vi" "Remote control"(FALSE ("Remote control")) -> ()
            n932 = global write "Dynamic_call_global.ph.vi" "Initial Plug Ins Extra"(w1485) -> ()
          }
          frame True {
          }
        }
        n933 = global write "Meas_global.vi" "Error handler Log"("") -> ()
      }
      frame #29 {
        # "Making Sure the Initial Plugin have stopped running"
        n934 = global read "Meas_global.vi" "Post Process"() -> (w1499:T2)
        n935 = case shown="\"Take New Data\"" w1499 {
          frame "Take New Data" {
            n936 = global read "Dynamic_call_global.ph.vi" "Initial Plug Ins Extra"() -> (w1503:string[])
            n937 = global read "Dynamic_call_global.ph.vi" "Initial Plug Ins"() -> (w1502:string[])
            n938 = Build Array (concatenate)(w1503, w1502) -> (w1500:string[])
            n939 = Empty Array?(array=w1500) -> (empty?=w1501:bool)
            n940 = case shown="False" w1501 {
              tunnel: w1500 -> [w1504 _]
              frame False {
                n941 = while {
                  tunnel: w1504 -> [w1507]
                  stop <- w1505 continue-if-true
                  n942 = for {
                    tunnel: w1507 -> [w1513] mode=indexing
                    tunnel: [w1513] -> w1506
                    tunnel: [w1512] -> w1505
                    stop <- w1512 stop-if-true
                    n943 = Open VI Reference(vi path=w1513) -> (vi reference=w1516:refnum<vi>, error out=w1517:errorcluster)  [unwired: 1 in, 4 out]
                    n944 = property class="VI"(reference=w1516, error in=w1517) -> (reference out=w1518:refnum<vi>, error out=w1519:errorcluster, "Execution:State"=w1515:T11)
                    n945 = Greater?(x=w1515, y=T11."Idle") -> (0:w1512:bool)
                    n946 = Close Reference(reference=w1518, error in (no error)=w1519) -> ()  [unwired: 1 out]
                  }
                  n947 = case shown="True" w1505 {
                    tunnel: w1506 -> [_ w1510]
                    frame False {
                    }
                    frame True {
                      n948 = Format Into String(format string="Waiting for %s to complete", w1510) -> (resulting string=w1508:string)  [unwired: 2 in, 1 out]
                      n949 = call "Wait_Seconds_with_display_Simple.vi"("Message"=w1508, "Seconds to wait"=2.0) -> ()  [unwired: 1 in, 1 out]
                    }
                  }
                }
              }
              frame True {
              }
            }
          }
          frame "Post Process Raw Data File" {
          }
        }
      }
      frame #30 {
        w1520 = FALSE
        n950 = local write "stop"(w1520) -> ()
        n951 = global write "Meas_global.vi" "Don't Process"(w1520) -> ()
      }
    }
  }
